vi "TEST.vi"() -> ()   [LabVIEW 2021]
uses:
  Control 4.ctl
  TEST ENNUM.ctl
  <vilib>/Utility/miscctls.llb/LVPointTypeDef.ctl
  Settings page.vi
  Exit Variable.vi
  <vilib>/Instr/_visa.llb/VISA Configure Serial Port (Instr).vi
  <vilib>/Utility/config.llb/Write Key (Double).vi
  <vilib>/Utility/file.llb/Write Delimited Spreadsheet (string).vi
  <vilib>/Utility/config.llb/NI_LVConfig.lvlib
  <userlib>/_OpenG.lib/string/string.llb/openg_string.lvlib
panel:
  out "Boolean":bool
  out "read buffer":string
  out "x/y":dbl
  out "output cluster":T1={"VISA resource name"="COM5", "MODE"="", "PP 1"=0, "PP 2"=0, "PP 3"=0, "PP 4"=0, "PP 5"=0, "PP 6"=0, "PP 7"=0, "PP 8"=0, "PP 9"=0, "PP 10"=0, "CH  PASS  1"=FALSE, "CH  PASS 2"=FALSE, "CH  PASS 3"=FALSE, "CH  PASS 4"=FALSE, "CH  PASS 5"=FALSE, "CH  PASS 6"=FALSE, "CH  PASS 7"=FALSE, "CH  PASS 8"=FALSE, "CH  PASS 9"=FALSE, "CH  PASS 10"=FALSE, "CH  FAIL 1"=FALSE, "CH  FAIL 2"=FALSE, "CH  FAIL 3"=FALSE, "CH  FAIL 4"=FALSE, "CH  FAIL 5"=FALSE, "CH  FAIL 6"=FALSE, "CH  FAIL 7"=FALSE, "CH  FAIL 8"=FALSE, "CH  FAIL 9"=FALSE, "CH  FAIL 10"=FALSE, "RES VALUE 1"=0.0, "RES VALUE 2"=0.0, "RES VALUE 3"=0.0, "RES VALUE 4"=0.0, "RES VALUE 5"=0.0, "RES VALUE 6"=0.0, "RES VALUE 7"=0.0, "RES VALUE 8"=0.0, "RES VALUE 9"=0.0, "RES VALUE 10"=0.0, "SET VALUE 1"=0.0, "SET VALUE 2"=0.0, "SET VALUE 3"=0.0, "SET VALUE 4"=0.0, "SET VALUE 5"=0.0, "SET VALUE 6"=0.0, "SET VALUE 7"=0.0, "SET VALUE 8"=0.0, "SET VALUE 9"=0.0, "SET VALUE 10"=0.0, "TOL 1"=0.0, "TOL 2"=0.0, "TOL 3"=0.0, "TOL 4"=0.0, "TOL 5"=0.0, "TOL 6"=0.0, "TOL 7"=0.0, "TOL 8"=0.0, "TOL 9"=0.0, "TOL 10"=0.0, "START BIT"=0, "CH1 MIN TOL"=0.0, "CH2 MIN TOL "=0.0, "CH3 MIN TOL "=0.0, "CH4 MIN TOL "=0.0, "CH5 MIN TOL "=0.0, "CH6 MIN TOL "=0.0, "CH7 MIN TOL  "=0.0, "CH8 MIN TOL  "=0.0, "CH9 MIN TOL   "=0.0, "CH10 MIN TOL   "=0.0, "CH1 MAX TOL "=0.0, "CH2 MAX TOL  "=0.0, "CH3 MAX TOL  "=0.0, "CH4 MAX TOL "=0.0, "CH5 MAX TOL  "=0.0, "CH6 MAX TOL  "=0.0, "CH7 MAX TOL   "=0.0, "CH8 MAX TOL  "=0.0, "CH9 MAX TOL    "=0.0, "CH10 MAX TOL   "=0.0} {"PP 10" format="%_1f"}
  in  "appended path":path
  out "Printer":bool
  out "Part ID":string
  out "Printer Command":string
  out "TETS TYPE":string
  out "TETS MODE":string
  in  "Exit Button":bool
  in  "SETTINGS BUTTON 2":bool
  out "Communication Status":bool
  out "CH 1 FAIL":bool
  out "CH 10 FAIL":bool
  out "CH 10  PASS":bool
  out "CH 5 FAIL":bool
  out "CH 5 PASS":bool
  out "CH 4 FAIL":bool
  out "CH 4 PASS":bool
  out "CH 9 FAIL":bool
  out "CH 9 PASS":bool
  out "CH 8 FAIL":bool
  out "CH 8 PASS":bool
  out "CH 3 FAIL":bool
  out "CH 3 PASS":bool
  out "CH 2 FAIL":bool
  out "CH 2 PASS":bool
  out "CH 7 FAIL":bool
  out "CH 7 PASS":bool
  out "CH 6 FAIL":bool
  out "CH 6 PASS":bool
  out "CH 1 PASS":bool
  out "CH 10 RES VAL":string
  out "CH 10 STATUS":string
  out "CH 9 RES VAL":string
  out "CH 9 STATUS":string
  out "CH 8 RES VAL":string
  out "CH 8 STATUS":string
  out "CH 7 RES VAL":string
  out "CH 7 STATUS":string
  out "CH 6 RES VAL":string
  out "CH 6 STATUS":string
  out "CH 5 RES VAL":string
  out "CH 5 STATUS":string
  out "CH 4 RES VAL":string
  out "CH 4 STATUS":string
  out "CH 3 RES VAL":string
  out "CH 3 STATUS":string
  out "CH 2 RES VAL":string
  out "CH 2 STATUS":string
  out "Cancel Button":bool
  out "CH 1 RES VAL":string
  out "CH1 STATUS":string
  # "EOL TEST BENCH FOR THERMISTOR"
  # "Communication Status"
  # "Printer Communication Status"
  # "CHANNEL 5"
  # "CHANNEL 3"
  # "CHANNEL 4"
  # "CHANNEL 1"
  # "CHANNEL 2"
  # "STATUS"
  # "STATUS"
  # "STATUS"
  # "STATUS"
  # "STATUS"
  # "k Ohm"
  # "k Ohm"
  # "RESISTANCE VALUE"
  # "RESISTANCE VALUE"
  # "RESISTANCE VALUE"
  # "k Ohm"
  # "RESISTANCE VALUE"
  # "k Ohm"
  # "RESISTANCE VALUE"
  # "k Ohm"
  # "PASS"
  # "FAIL"
  # "PASS"
  # "FAIL"
  # "PASS"
  # "FAIL"
  # "PASS"
  # "FAIL"
  # "PASS"
  # "FAIL"
  # "QR DATA"
  # "CHANNEL 7"
  # "CHANNEL 6"
  # "CHANNEL 10"
  # "CHANNEL 8"
  # "CHANNEL 9"
  # "STATUS"
  # "STATUS"
  # "STATUS"
  # "STATUS"
  # "STATUS"
  # "RESISTANCE VALUE"
  # "RESISTANCE VALUE"
  # "k Ohm"
  # "RESISTANCE VALUE"
  # "Control 4.ctlk Ohm"
  # "RESISTANCE VALUE"
  # "k Ohm"
  # "k Ohm"
  # "RESISTANCE VALUE"
  # "k Ohm"
  # "PASS"
  # "FAIL"
  # "PASS"
  # "FAIL"
  # "PASS"
  # "FAIL"
  # "PASS"
  # "FAIL"
  # "PASS"
  # "FAIL"
  # "MODE :"
  # "TEST TYPE :"
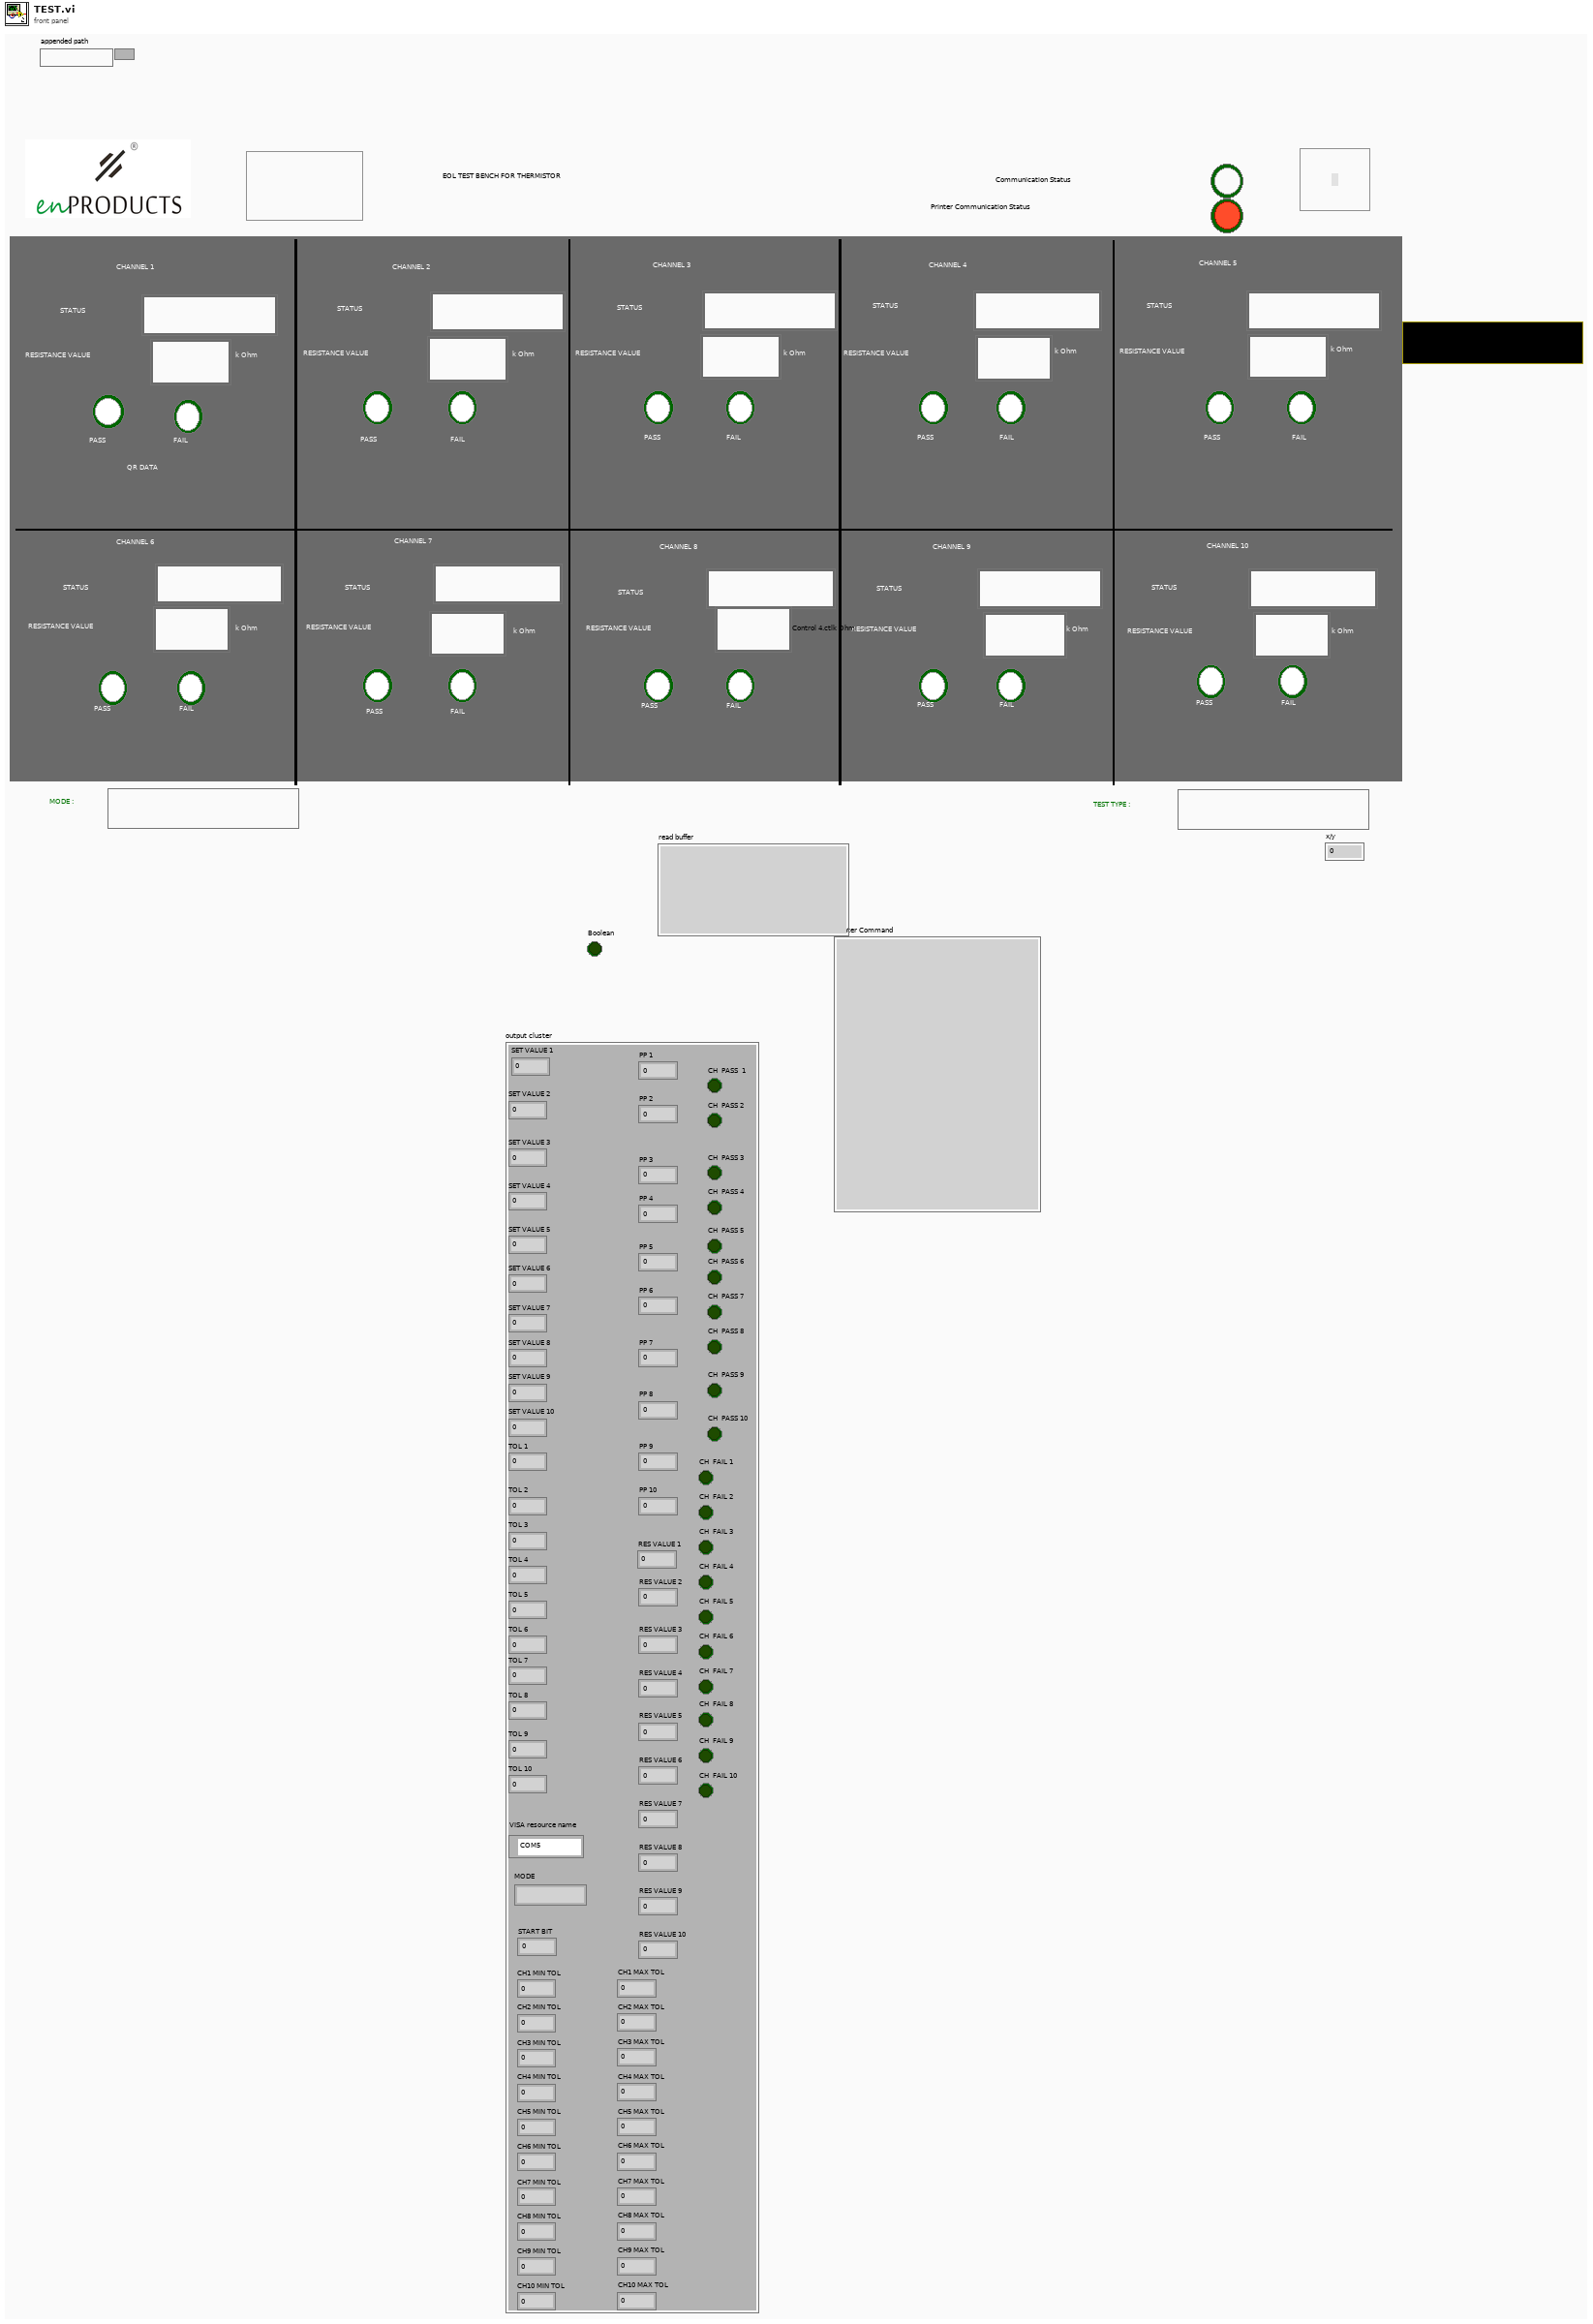
[diagram p1: front panel]
types:
  T1 = typedef "Control 4.ctl" = cluster{"VISA resource name":refnum<visa-resource-name>, "MODE":string, "PP 1":i32, "PP 2":i32, "PP 3":i32, "PP 4":i32, "PP 5":i32, "PP 6":i32, "PP 7":i32, "PP 8":i32, "PP 9":i32, "PP 10":i32, "CH  PASS  1":bool, "CH  PASS 2":bool, "CH  PASS 3":bool, "CH  PASS 4":bool, "CH  PASS 5":bool, "CH  PASS 6":bool, "CH  PASS 7":bool, "CH  PASS 8":bool, "CH  PASS 9":bool, "CH  PASS 10":bool, "CH  FAIL 1":bool, "CH  FAIL 2":bool, "CH  FAIL 3":bool, "CH  FAIL 4":bool, "CH  FAIL 5":bool, "CH  FAIL 6":bool, "CH  FAIL 7":bool, "CH  FAIL 8":bool, "CH  FAIL 9":bool, "CH  FAIL 10":bool, "RES VALUE 1":dbl, "RES VALUE 2":dbl, "RES VALUE 3":dbl, "RES VALUE 4":dbl, "RES VALUE 5":dbl, "RES VALUE 6":dbl, "RES VALUE 7":dbl, "RES VALUE 8":dbl, "RES VALUE 9":dbl, "RES VALUE 10":dbl, "SET VALUE 1":dbl, "SET VALUE 2":dbl, "SET VALUE 3":dbl, "SET VALUE 4":dbl, "SET VALUE 5":dbl, "SET VALUE 6":dbl, "SET VALUE 7":dbl, "SET VALUE 8":dbl, "SET VALUE 9":dbl, "SET VALUE 10":dbl, "TOL 1":dbl, "TOL 2":dbl, "TOL 3":dbl, "TOL 4":dbl, "TOL 5":dbl, "TOL 6":dbl, "TOL 7":dbl, "TOL 8":dbl, "TOL 9":dbl, "TOL 10":dbl, "START BIT":i32, "CH1 MIN TOL":dbl, "CH2 MIN TOL ":dbl, "CH3 MIN TOL ":dbl, "CH4 MIN TOL ":dbl, "CH5 MIN TOL ":dbl, "CH6 MIN TOL ":dbl, "CH7 MIN TOL  ":dbl, "CH8 MIN TOL  ":dbl, "CH9 MIN TOL   ":dbl, "CH10 MIN TOL   ":dbl, "CH1 MAX TOL ":dbl, "CH2 MAX TOL  ":dbl, "CH3 MAX TOL  ":dbl, "CH4 MAX TOL ":dbl, "CH5 MAX TOL  ":dbl, "CH6 MAX TOL  ":dbl, "CH7 MAX TOL   ":dbl, "CH8 MAX TOL  ":dbl, "CH9 MAX TOL    ":dbl, "CH10 MAX TOL   ":dbl}
  T2 = typedef "LVPointTypeDef.ctl" = cluster{"Horizontal":i16, "Vertical":i16}
  T3 = typedef "TEST ENNUM.ctl" = enum16{"TIMEOUT", "INITIALIZE", "CH SELECTION", "VALIDATING", "RESULT", "LED_SEQ", "READY TO PRINT", "REPORT ", "PART PRESENCE CHECKING"}
  T4 = typedef "NI_LVConfig.lvlib/Config Data RefNum.ctl" = refnum<k1>
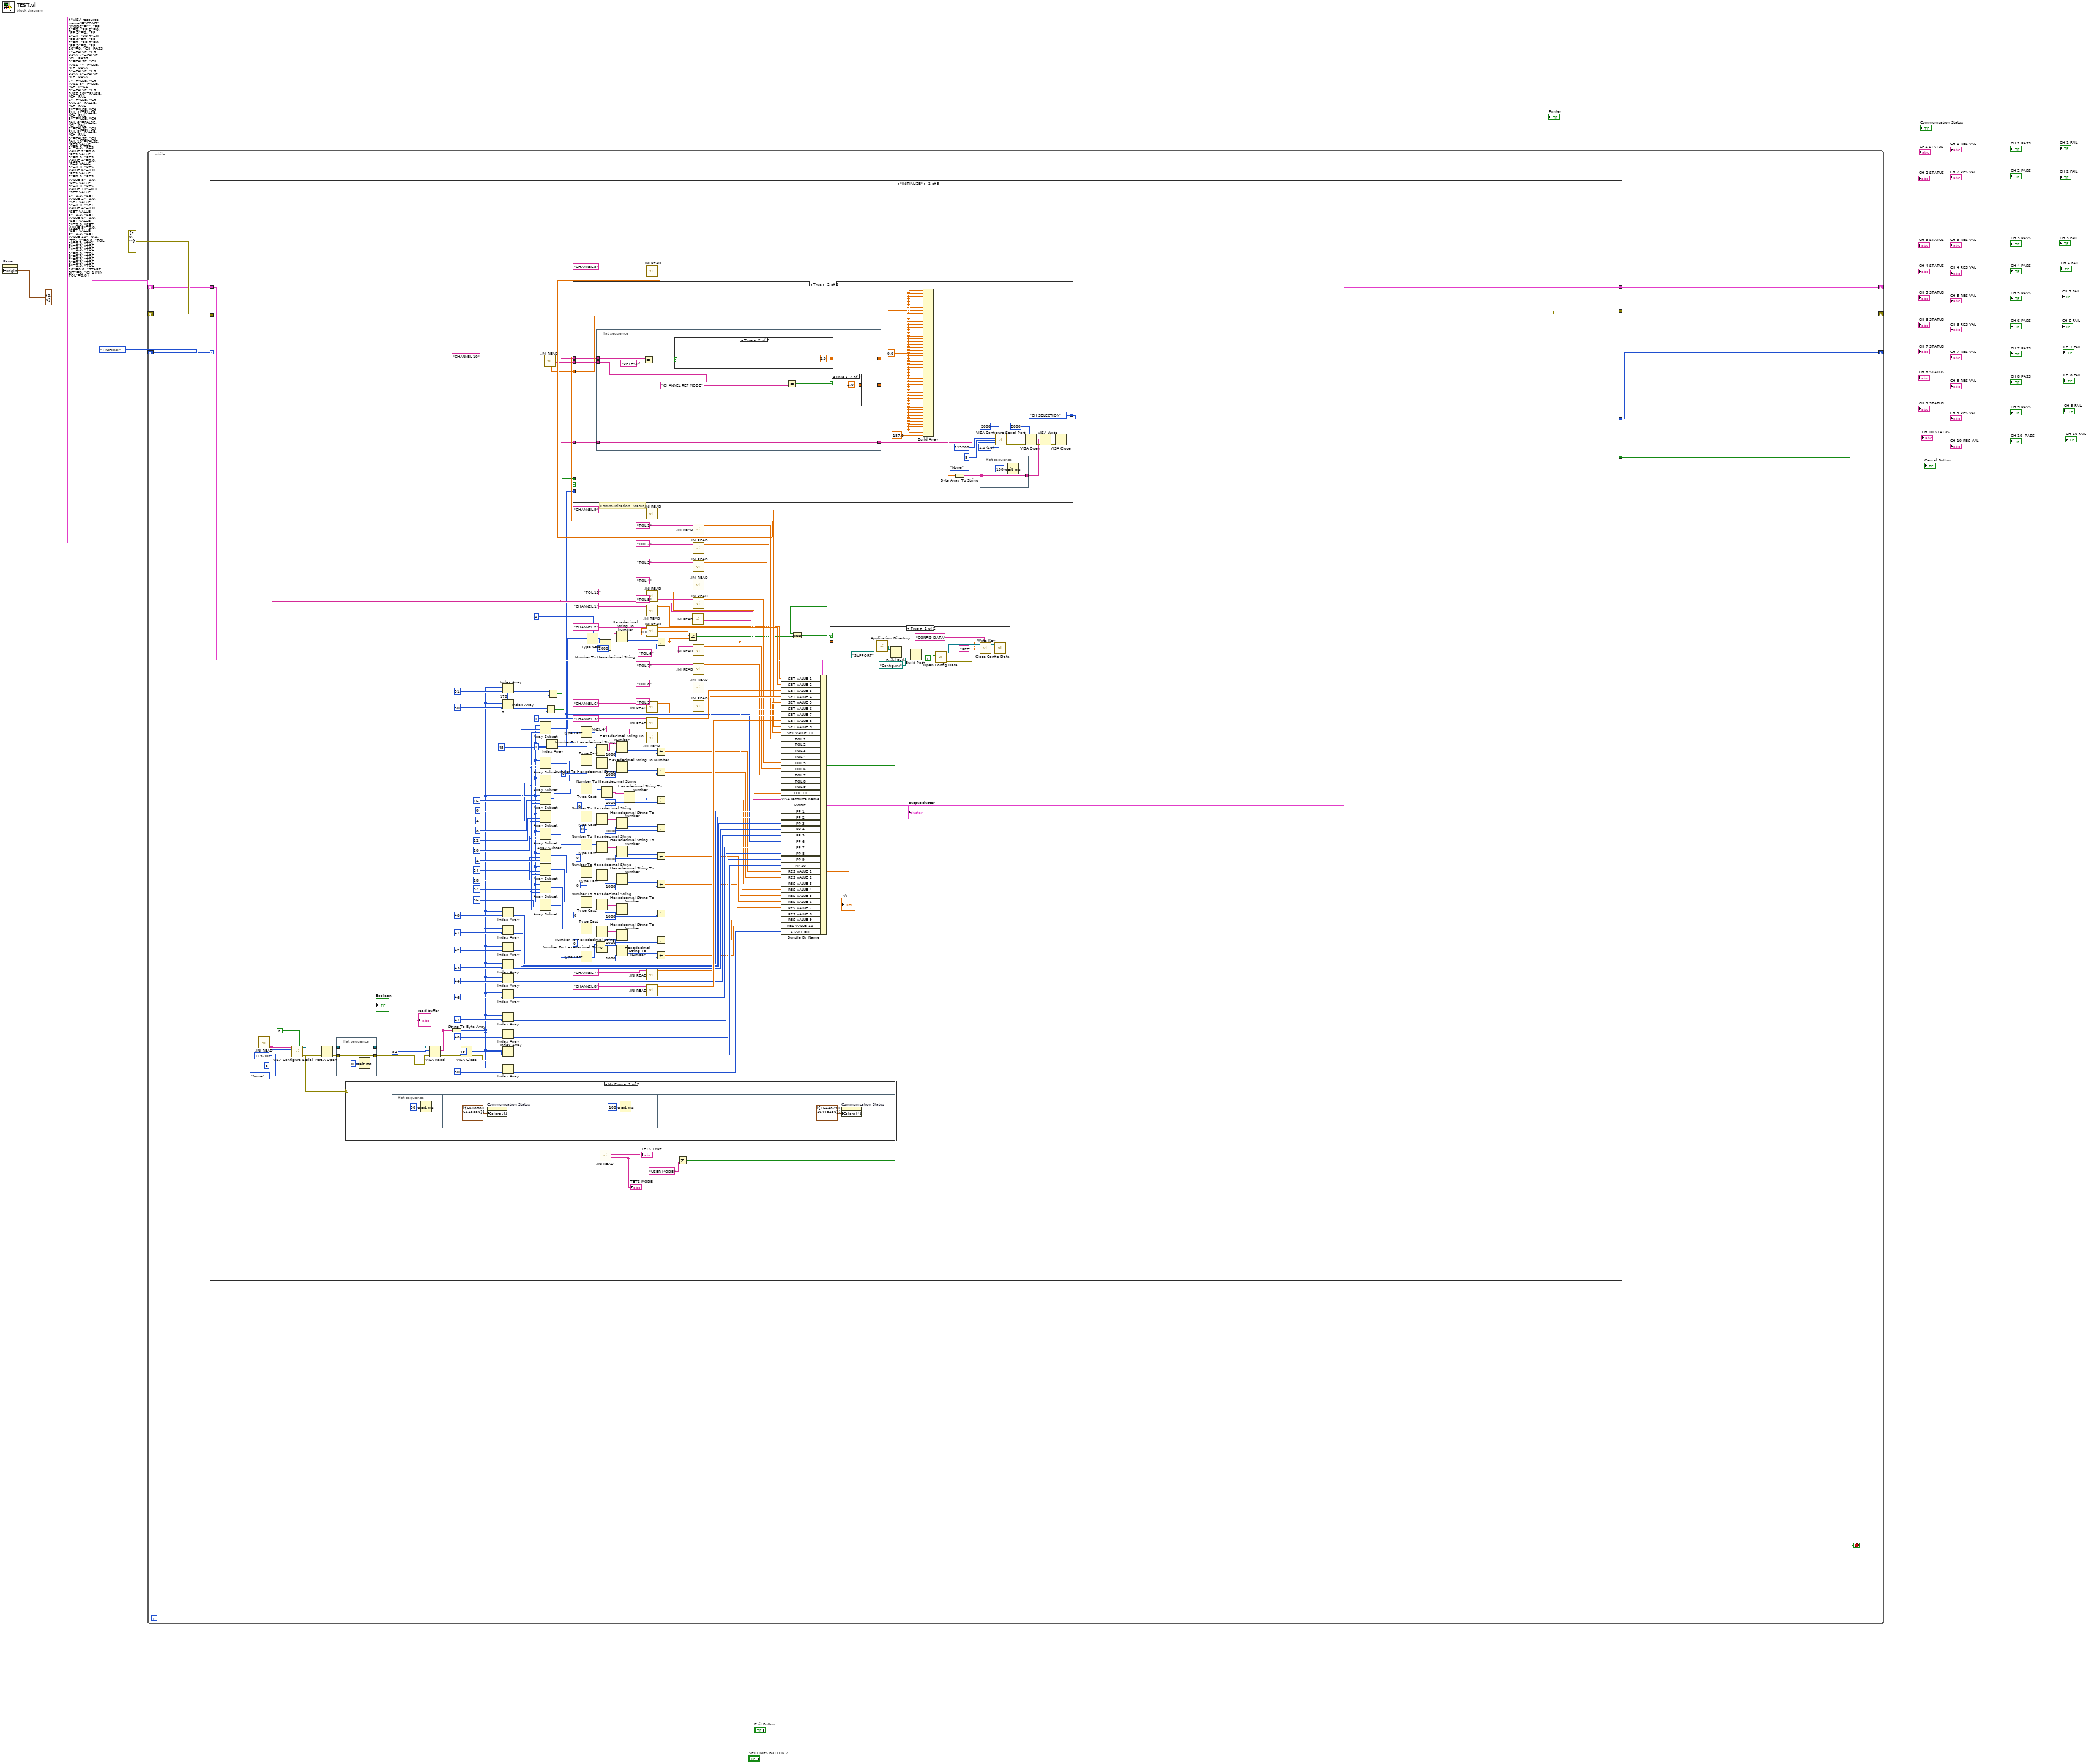
[diagram p0: block diagram]
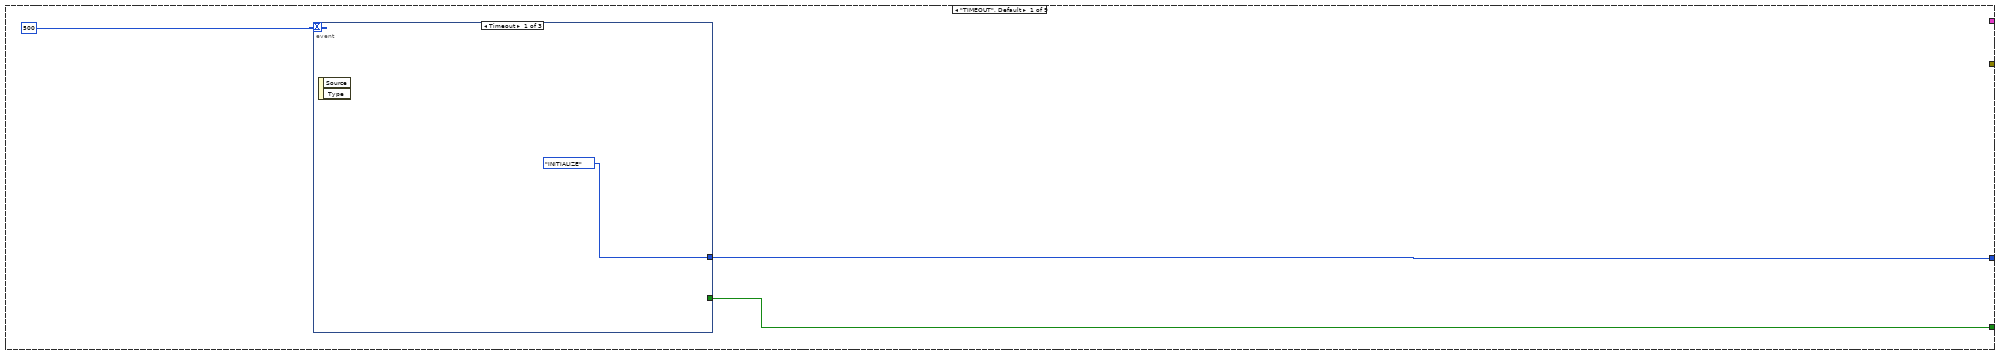
[diagram p2: hidden frame]
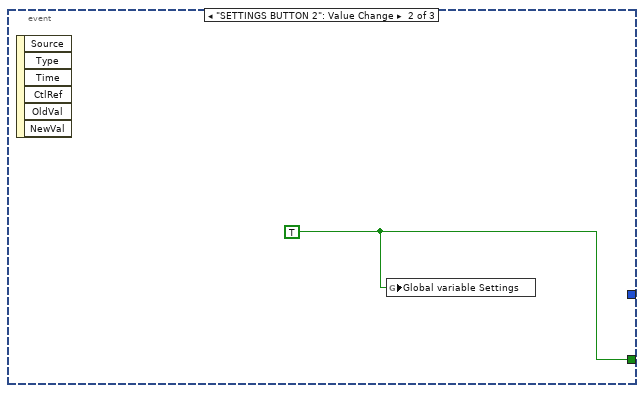
[diagram p3: hidden frame]
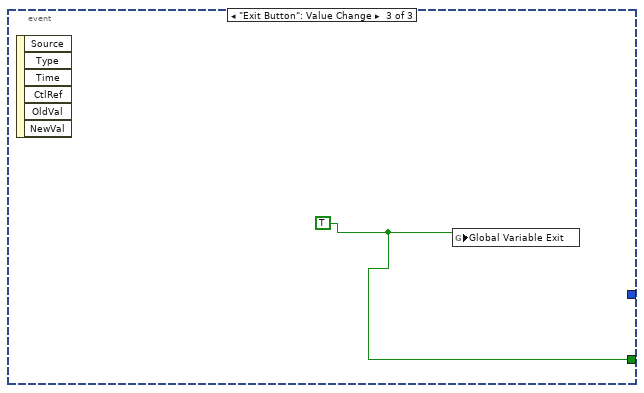
[diagram p4: hidden frame]
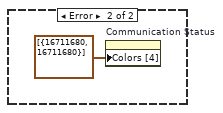
[diagram p6: hidden frame]
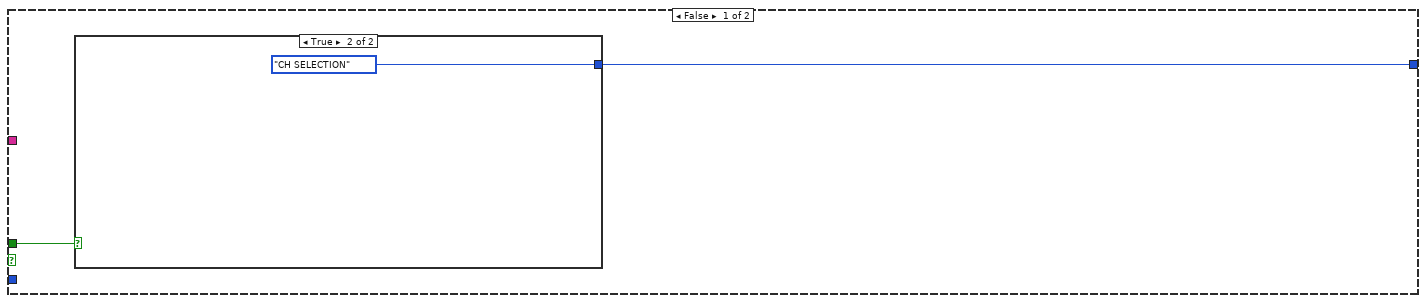
[diagram p7: hidden frame]
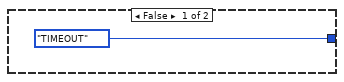
[diagram p8: hidden frame]
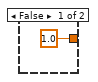
[diagram p9: hidden frame]
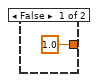
[diagram p10: hidden frame]
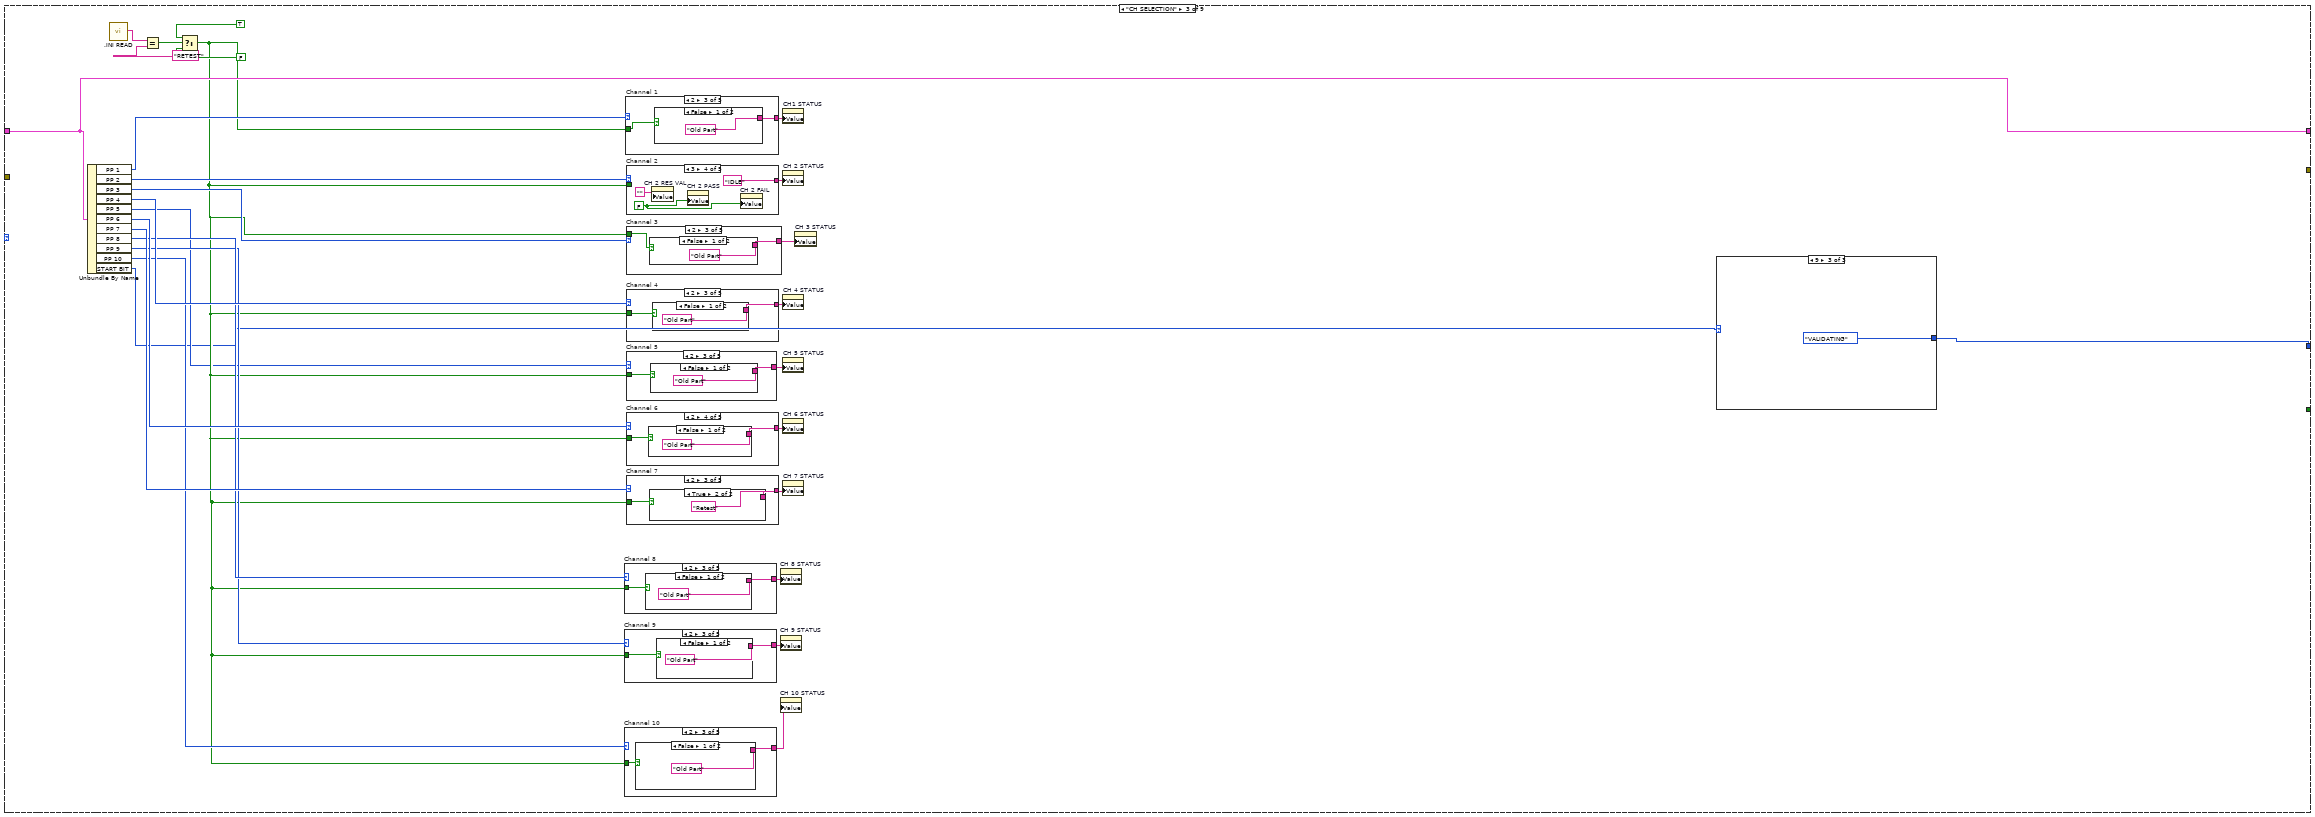
[diagram p11: hidden frame]
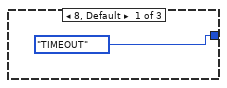
[diagram p12: hidden frame]
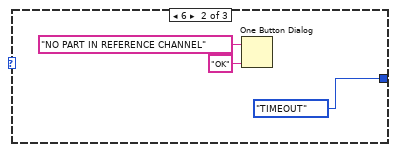
[diagram p13: hidden frame]
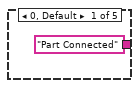
[diagram p14: hidden frame]
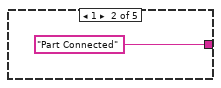
[diagram p15: hidden frame]
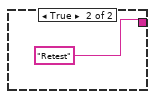
[diagram p16: hidden frame]
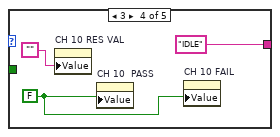
[diagram p17: hidden frame]
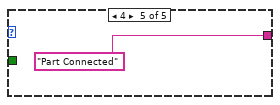
[diagram p18: hidden frame]
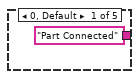
[diagram p19: hidden frame]
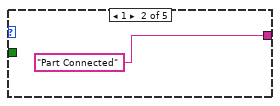
[diagram p20: hidden frame]
diagram:
  n1 = property on="Pane" class="Pane"("Origin"=T2 {"Horizontal"=0, "Vertical"=0}) -> ()  [unwired: 2 in, 2 out]
  n2 = while {
    shift-right: [w10] -> _
    shift-left: TEST_ENNUM."TIMEOUT" -> [w11]
    shift-right: [w9] -> _
    shift-left: T1 {"VISA resource name"="COM5", "MODE"="", "PP 1"=0, "PP 2"=0, "PP 3"=0, "PP 4"=0, "PP 5"=0, "PP 6"=0, "PP 7"=0, "PP 8"=0, "PP 9"=0, "PP 10"=0, "CH  PASS  1"=FALSE, "CH  PASS 2"=FALSE, "CH  PASS 3"=FALSE, "CH  PASS 4"=FALSE, "CH  PASS 5"=FALSE, "CH  PASS 6"=FALSE, "CH  PASS 7"=FALSE, "CH  PASS 8"=FALSE, "CH  PASS 9"=FALSE, "CH  PASS 10"=FALSE, "CH  FAIL 1"=FALSE, "CH  FAIL 2"=FALSE, "CH  FAIL 3"=FALSE, "CH  FAIL 4"=FALSE, "CH  FAIL 5"=FALSE, "CH  FAIL 6"=FALSE, "CH  FAIL 7"=FALSE, "CH  FAIL 8"=FALSE, "CH  FAIL 9"=FALSE, "CH  FAIL 10"=FALSE, "RES VALUE 1"=0.0, "RES VALUE 2"=0.0, "RES VALUE 3"=0.0, "RES VALUE 4"=0.0, "RES VALUE 5"=0.0, "RES VALUE 6"=0.0, "RES VALUE 7"=0.0, "RES VALUE 8"=0.0, "RES VALUE 9"=0.0, "RES VALUE 10"=0.0, "SET VALUE 1"=0.0, "SET VALUE 2"=0.0, "SET VALUE 3"=0.0, "SET VALUE 4"=0.0, "SET VALUE 5"=0.0, "SET VALUE 6"=0.0, "SET VALUE 7"=0.0, "SET VALUE 8"=0.0, "SET VALUE 9"=0.0, "SET VALUE 10"=0.0, "TOL 1"=0.0, "TOL 2"=0.0, "TOL 3"=0.0, "TOL 4"=0.0, "TOL 5"=0.0, "TOL 6"=0.0, "TOL 7"=0.0, "TOL 8"=0.0, "TOL 9"=0.0, "TOL 10"=0.0, "START BIT"=0, "CH1 MIN TOL"=0.0, "CH2 MIN TOL "=0.0, "CH3 MIN TOL "=0.0, "CH4 MIN TOL "=0.0, "CH5 MIN TOL "=0.0, "CH6 MIN TOL "=0.0, "CH7 MIN TOL  "=0.0, "CH8 MIN TOL  "=0.0, "CH9 MIN TOL   "=0.0, "CH10 MIN TOL   "=0.0, "CH1 MAX TOL "=0.0, "CH2 MAX TOL  "=0.0, "CH3 MAX TOL  "=0.0, "CH4 MAX TOL "=0.0, "CH5 MAX TOL  "=0.0, "CH6 MAX TOL  "=0.0, "CH7 MAX TOL   "=0.0, "CH8 MAX TOL  "=0.0, "CH9 MAX TOL    "=0.0, "CH10 MAX TOL   "=0.0} ("Cluster") -> [w7]
    shift-right: [w8] -> _
    shift-left: errorcluster {"status"=FALSE, "code"=0, "source"=""} ("error out") -> [w6]
    stop <- w5 stop-if-true
    n3 = case shown="\"INITIALIZE\"" w11 {
      tunnel: [w13 w55 w265 TEST_ENNUM."RESULT" TEST_ENNUM."LED_SEQ" TEST_ENNUM."READY TO PRINT" TEST_ENNUM."REPORT " TEST_ENNUM."TIMEOUT" _] -> w10
      tunnel: w7 -> [_ w139 w274 w421 w641 w860 w1021 w1032 _]
      tunnel: [_ w140 w274 w534 w641 w860 _ _ _] -> w9
      tunnel: [_ w59 _ _ _ w858 _ _ _] -> w8
      tunnel: w6 -> [_ _ _ _ _ _ _ _ _]
      tunnel: [w12 _ _ _ _ _ _ _ _] -> w5
      frame "TIMEOUT", Default {
        n4 = event shown="[0] Timeout" {
          selector: _ -> [_ _ _]
          dyn-events: _ -> [_ _ _]
          timeout: 500 -> [_ _ _]
          tunnel: [_ w16 w17] -> w12
          tunnel: [TEST_ENNUM."INITIALIZE" _ _] -> w13
          event Timeout {
            n5 = event-data() -> ()  [unwired: 1 in, 2 out]
          }
          event "SETTINGS BUTTON 2": Value Change {
            w16 = TRUE
            n6 = event-data() -> ()  [unwired: 1 in, 6 out]
            n7 = global write "Settings page.vi" "Global variable Settings"(w16) -> ()
          }
          event "Exit Button": Value Change {
            w17 = TRUE
            n8 = event-data() -> ()  [unwired: 1 in, 6 out]
            n9 = global write "Exit Variable.vi" "Global Variable Exit"(w17) -> ()
          }
        }
      }
      frame "INITIALIZE" {
        w137 = 4 ("length")
        # "Communication  Status"
        n10 = call ".INI READ.vi"() -> ("COM"=w56:string)  [unwired: 4 in, 7 out]
        n11 = call-poly "VISA Configure Serial Port"("VISA resource name"=w56, "Enable Termination\nChar (T)"=FALSE ("Enable Termination\nChar (T)"), "baud rate (9600)"=u32 115200, "data bits (8)"=u16 8, "parity (0:none)"=enum16{"None", "Odd", "Even", "Mark", "Space"}."None") -> ("VISA resource name out"=w47:refnum<visa-resource-name>, "error out"=w61:errorcluster)  [unwired: 9 in]
        n12 = VISA Open(error in (no error)=w61, VISA resource name=w47) -> (VISA resource name=w42:refnum<visa-resource-name>, error out=w44:errorcluster)  [unwired: 3 in]
        n13 = flat-sequence {
          tunnel: [w215] -> w21
          tunnel: w44 -> [w215]
          tunnel: [w214] -> w43
          tunnel: w42 -> [w214]
          frame #0 {
            n14 = Wait (ms)(milliseconds to wait=u32 0) -> ()  [unwired: 1 out]
          }
        }
        n15 = case shown="No Error" w61 {
          frame No Error {
            n16 = flat-sequence {
              frame #0 {
                n17 = Wait (ms)(milliseconds to wait=u32 50) -> ()  [unwired: 1 out]
              }
              frame #1 {
                n18 = property on="Communication Status" class="Bool (strict)"("Colors [4]"=cluster{u32, u32}[] [{6618880, 6618880}]) -> ()  [unwired: 2 in, 2 out]
              }
              frame #2 {
                n19 = Wait (ms)(milliseconds to wait=u32 100) -> ()  [unwired: 1 out]
              }
              frame #3 {
                n20 = property on="Communication Status" class="Bool (strict)"("Colors [4]"=cluster{u32, u32}[] [{16448250, 16448250}]) -> ()  [unwired: 2 in, 2 out]
              }
            }
          }
          frame Error {
            n21 = property on="Communication Status" class="Bool (strict)"("Colors [4]"=cluster{u32, u32}[] [{16711680, 16711680}]) -> ()  [unwired: 2 in, 2 out]
          }
        }
        n22 = VISA Read(VISA resource name=w43, byte count=u32 52, error in (no error)=w21) -> (VISA resource name out=w19:refnum<visa-resource-name>, read buffer=w20:string, error out=w18:errorcluster)  [unwired: 1 out]
        "read buffer" <- w20
        n23 = String To Byte Array(string=w20) -> (unsigned byte array=w34:u8[])
        n24 = VISA Close(VISA resource name=w19, error in (no error)=w18) -> (error out=w59:errorcluster)
        n25 = Index Array(array=w34, index=51) -> (element=w57:u8)
        n26 = Index Array(array=w34, index=50) -> (element=w52:u8)
        n27 = Index Array(array=w34, index=40) -> (element=w149:u8)
        n28 = Index Array(array=w34, index=41) -> (element=w148:u8)
        n29 = Index Array(array=w34, index=42) -> (element=w147:u8)
        n30 = Index Array(array=w34, index=43) -> (element=w146:u8)
        n31 = Index Array(array=w34, index=44) -> (element=w145:u8)
        n32 = Index Array(array=w34, index=46) -> (element=w144:u8)
        n33 = Index Array(array=w34, index=47) -> (element=w143:u8)
        n34 = Index Array(array=w34, index=48) -> (element=w142:u8)
        n35 = Index Array(array=w34, index=49) -> (element=w141:u8)
        n36 = Index Array(array=w34, index=50) -> (element=w60:u8)
        n37 = Array Subset(array=w34, index=16, length=w137) -> (w109:u8[])
        n38 = Array Subset(array=w34, index=0, length=w137) -> (w24:u8[])
        n39 = Array Subset(array=w34, index=4, length=w137) -> (w116:u8[])
        n40 = Array Subset(array=w34, index=8, length=w137) -> (w23:u8[])
        n41 = Array Subset(array=w34, index=12, length=w137) -> (w112:u8[])
        n42 = Array Subset(array=w34, index=20, length=w137) -> (w106:u8[])
        n43 = Array Subset(array=w34, index=24, length=w137) -> (w103:u8[])
        n44 = Array Subset(array=w34, index=28, length=w137) -> (w100:u8[])
        n45 = Array Subset(array=w34, index=32, length=w137) -> (w97:u8[])
        n46 = Array Subset(array=w34, index=36, length=w137) -> (w94:u8[])
        n47 = call ".INI READ.vi"("KEY"="CHANNEL 10") -> ("MODE"=w30:string, "TEST MODE"=w29:string, "OUT"=w181:dbl, "TIME"=w31:dbl)  [unwired: 3 in, 4 out]
        n48 = Equal?(x=w52, y=u8 8) -> (x = y?=w50:bool)
        n49 = Index Array(array=w34, index=45) -> (element=w32:u8)
        n50 = Equal?(x=w57, y=u8 170) -> (x = y?=w53:bool)
        n51 = case shown="True" w50 {
          tunnel: w56 -> [_ w229]
          tunnel: [w221 TEST_ENNUM."CH SELECTION"] -> w55
          tunnel: w53 -> [w222 _]
          tunnel: w32 -> [_ _]
          tunnel: w30 -> [_ w227]
          tunnel: w31 -> [_ w226]
          tunnel: w29 -> [_ w225]
          frame False {
            n52 = case shown="True" w222 {
              tunnel: [TEST_ENNUM."TIMEOUT" TEST_ENNUM."CH SELECTION"] -> w221
              frame False {
              }
              frame True {
              }
            }
          }
          frame True {
            w242 = u16 10 items=["1.0"=10, "1.5"=15, "2.0"=20] ("stop bits (10: 1 bit)")
            w233 = 0.0 ("element")
            n53 = flat-sequence {
              tunnel: [w256] -> w231
              tunnel: [w253] -> w230
              tunnel: w229 -> [w252]
              tunnel: [w252] -> w228
              tunnel: w227 -> [w251]
              tunnel: w225 -> [w250]
              frame #0 {
                n54 = Equal?(x=w250, y="RETEST") -> (x = y?=w257:bool)
                n55 = case shown="True" w257 {
                  tunnel: [1.0 ("element") 2.0 ("element")] -> w256
                  frame False {
                  }
                  frame True {
                  }
                }
                n56 = Equal?(x=w251, y="CHANNEL REF MODE") -> (x = y?=w254:bool)
                n57 = case shown="True" w254 {
                  tunnel: [1.0 ("element") 2.0 ("element")] -> w253
                  frame False {
                  }
                  frame True {
                  }
                }
              }
            }
            n58 = Build Array(w233, w233, w233, w233, w233, w233, w231, w230, w233, w226, w233, w233, w233, w233, w233, w233, w233, w233, w233, w233, w233, w233, w233, w233, w233, w233, w233, w233, w233, w233, w233, w233, w233, w233, w233, w233, w233, w233, w233, w233, w233, w233, w233, w233, w233, w233, w233, w233, w233, w233, w233, 187.0 ("element")) -> (w249:dbl[])
            n59 = Byte Array To String(unsigned byte array=w249) -> (string=w235:string)
            n60 = flat-sequence {
              tunnel: w235 -> [w264]
              tunnel: [w264] -> w234
              frame #0 {
                n61 = Wait (ms)(milliseconds to wait=u32 100) -> ()  [unwired: 1 out]
              }
            }
            n62 = call-poly "VISA Configure Serial Port"("VISA resource name"=w228, "timeout (10sec)"=u32 2000, "baud rate (9600)"=u32 115200, "data bits (8)"=u16 8, "parity (0:none)"=enum16{"None", "Odd", "Even", "Mark", "Space"}."None", "stop bits (10: 1 bit)"=w242) -> ("VISA resource name out"=w248:refnum<visa-resource-name>, "error out"=w247:errorcluster)  [unwired: 8 in]
            n63 = VISA Open(timeout (0)=u32 2000 ("VISA Open timeout (0)"), error in (no error)=w247, VISA resource name=w248) -> (VISA resource name=w241:refnum<visa-resource-name>, error out=w240:errorcluster)  [unwired: 2 in]
            n64 = VISA Write(VISA resource name=w241, write buffer=w234, error in (no error)=w240) -> (VISA resource name out=w238:refnum<visa-resource-name>, error out=w237:errorcluster)  [unwired: 1 out]
            n65 = VISA Close(VISA resource name=w238, error in (no error)=w237) -> ()  [unwired: 1 out]
          }
        }
        n66 = Type Cast(type=0 ("index"), x=w24) -> (*(type *) &x=w118:i32)
        n67 = Type Cast(type=0 ("index"), x=w116) -> (*(type *) &x=w115:i32)
        n68 = Type Cast(type=0 ("index"), x=w23) -> (*(type *) &x=w22:i32)
        n69 = Type Cast(type=0 ("index"), x=w112) -> (*(type *) &x=w111:i32)
        n70 = Type Cast(type=0 ("index"), x=w106) -> (*(type *) &x=w105:i32)
        n71 = Type Cast(type=0 ("index"), x=w103) -> (*(type *) &x=w102:i32)
        n72 = Type Cast(type=0 ("index"), x=w100) -> (*(type *) &x=w99:i32)
        n73 = Type Cast(type=0 ("index"), x=w97) -> (*(type *) &x=w96:i32)
        n74 = Type Cast(type=0 ("index"), x=w94) -> (*(type *) &x=w93:i32)
        n75 = Type Cast(type=0 ("index"), x=w109) -> (*(type *) &x=w108:i32)
        n76 = Number To Hexadecimal String(2:w118) -> (0:w117:string)  [unwired: 1 in]
        n77 = Number To Hexadecimal String(2:w115) -> (0:w114:string)  [unwired: 1 in]
        n78 = Number To Hexadecimal String(2:w111) -> (0:w110:string)  [unwired: 1 in]
        n79 = Number To Hexadecimal String(2:w105) -> (0:w104:string)  [unwired: 1 in]
        n80 = Number To Hexadecimal String(2:w102) -> (0:w101:string)  [unwired: 1 in]
        n81 = Number To Hexadecimal String(2:w99) -> (0:w98:string)  [unwired: 1 in]
        n82 = Number To Hexadecimal String(2:w96) -> (0:w95:string)  [unwired: 1 in]
        n83 = Number To Hexadecimal String(2:w93) -> (0:w92:string)  [unwired: 1 in]
        n84 = Number To Hexadecimal String(2:w108) -> (0:w107:string)  [unwired: 1 in]
        n85 = call ".INI READ.vi"() -> ("MODE"=w28:string, "TEST MODE"=→"TETS TYPE":string)  [unwired: 4 in, 6 out]
        "TETS MODE" <- w28
        n86 = Number To Hexadecimal String(2:w22) -> (0:w113:string)  [unwired: 1 in]
        n87 = Hexadecimal String To Number(string=w107) -> (number=w80:u32)  [unwired: 2 in, 1 out]
        n88 = Hexadecimal String To Number(string=w117) -> (number=w91:u32)  [unwired: 2 in, 1 out]
        n89 = Hexadecimal String To Number(string=w114) -> (number=w88:u32)  [unwired: 2 in, 1 out]
        n90 = Hexadecimal String To Number(string=w110) -> (number=w83:u32)  [unwired: 2 in, 1 out]
        n91 = Hexadecimal String To Number(string=w104) -> (number=w65:u32)  [unwired: 2 in, 1 out]
        n92 = Hexadecimal String To Number(string=w101) -> (number=w77:u32)  [unwired: 2 in, 1 out]
        n93 = Hexadecimal String To Number(string=w98) -> (number=w74:u32)  [unwired: 2 in, 1 out]
        n94 = Hexadecimal String To Number(string=w95) -> (number=w71:u32)  [unwired: 2 in, 1 out]
        n95 = Hexadecimal String To Number(string=w92) -> (number=w68:u32)  [unwired: 2 in, 1 out]
        n96 = Hexadecimal String To Number(string=w113) -> (number=w86:u32)  [unwired: 2 in, 1 out]
        n97 = call ".INI READ.vi"("KEY"="CHANNEL 5") -> ("OUT"=w186:dbl)  [unwired: 3 in, 7 out]
        n98 = call ".INI READ.vi"("KEY"="CHANNEL 9") -> ("OUT"=w182:dbl)  [unwired: 3 in, 7 out]
        n99 = call ".INI READ.vi"("KEY"="TOL 10") -> ("OUT"=w161:dbl)  [unwired: 3 in, 7 out]
        n100 = call ".INI READ.vi"("KEY"="CHANNEL 1") -> ("OUT"=w39:dbl)  [unwired: 3 in, 7 out]
        n101 = call ".INI READ.vi"("KEY"="CHANNEL 2") -> ("OUT"=w189:dbl)  [unwired: 3 in, 7 out]
        n102 = call ".INI READ.vi"("KEY"="CHANNEL 6") -> ("OUT"=w185:dbl)  [unwired: 3 in, 7 out]
        n103 = call ".INI READ.vi"("KEY"="CHANNEL 3") -> ("OUT"=w188:dbl)  [unwired: 3 in, 7 out]
        n104 = call ".INI READ.vi"("KEY"="CHANNEL 4") -> ("OUT"=w187:dbl)  [unwired: 3 in, 7 out]
        n105 = call ".INI READ.vi"("KEY"="CHANNEL 7") -> ("OUT"=w184:dbl)  [unwired: 3 in, 7 out]
        n106 = call ".INI READ.vi"("KEY"="CHANNEL 8") -> ("OUT"=w183:dbl)  [unwired: 3 in, 7 out]
        n107 = Divide(x=w91, y=u32 1000) -> (x/y=w26:dbl)
        "x/y" <- w26
        n108 = Divide(x=w88, y=u32 1000) -> (x/y=w87:dbl)
        n109 = Divide(x=w86, y=u32 1000) -> (x/y=w84:dbl)
        n110 = Divide(x=w83, y=u32 1000) -> (x/y=w81:dbl)
        n111 = Divide(x=w65, y=u32 1000) -> (x/y=w78:dbl)
        n112 = Divide(x=w77, y=u32 1000) -> (x/y=w75:dbl)
        n113 = Divide(x=w74, y=u32 1000) -> (x/y=w72:dbl)
        n114 = Divide(x=w71, y=u32 1000) -> (x/y=w69:dbl)
        n115 = Divide(x=w68, y=u32 1000) -> (x/y=w63:dbl)
        n116 = Divide(x=w80, y=u32 1000) -> (x/y=w33:dbl)
        n117 = Not Equal?(x=w28, y="USER MODE") -> (x != y?=w36:bool)
        n118 = Not Equal?(x=0.0, y=w33) -> (x != y?=w37:bool)
        n119 = call ".INI READ.vi"() -> ("MODE"=w160:string)  [unwired: 4 in, 7 out]
        n120 = call ".INI READ.vi"("KEY"="TOL 1") -> ("OUT"=w170:dbl)  [unwired: 3 in, 7 out]
        n121 = call ".INI READ.vi"("KEY"="TOL 2") -> ("OUT"=w169:dbl)  [unwired: 3 in, 7 out]
        n122 = call ".INI READ.vi"("KEY"="TOL 3") -> ("OUT"=w168:dbl)  [unwired: 3 in, 7 out]
        n123 = call ".INI READ.vi"("KEY"="TOL 4") -> ("OUT"=w167:dbl)  [unwired: 3 in, 7 out]
        n124 = call ".INI READ.vi"("KEY"="TOL 5") -> ("OUT"=w166:dbl)  [unwired: 3 in, 7 out]
        n125 = call ".INI READ.vi"("KEY"="TOL 6") -> ("OUT"=w165:dbl)  [unwired: 3 in, 7 out]
        n126 = call ".INI READ.vi"("KEY"="TOL 7") -> ("OUT"=w164:dbl)  [unwired: 3 in, 7 out]
        n127 = call ".INI READ.vi"("KEY"="TOL 8") -> ("OUT"=w163:dbl)  [unwired: 3 in, 7 out]
        n128 = call ".INI READ.vi"("KEY"="TOL 9") -> ("OUT"=w162:dbl)  [unwired: 3 in, 7 out]
        n129 = Bundle By Name(cluster=w139, "SET VALUE 1"=w39, "SET VALUE 2"=w189, "SET VALUE 3"=w188, "SET VALUE 4"=w187, "SET VALUE 5"=w186, "SET VALUE 6"=w185, "SET VALUE 7"=w184, "SET VALUE 8"=w183, "SET VALUE 9"=w182, "SET VALUE 10"=w181, "TOL 1"=w170, "TOL 2"=w169, "TOL 3"=w168, "TOL 4"=w167, "TOL 5"=w166, "TOL 6"=w165, "TOL 7"=w164, "TOL 8"=w163, "TOL 9"=w162, "TOL 10"=w161, "VISA resource name"=w56, "MODE"=w160, "PP 1"=w149, "PP 2"=w148, "PP 3"=w147, "PP 4"=w146, "PP 5"=w145, "PP 6"=w32, "PP 7"=w144, "PP 8"=w143, "PP 9"=w142, "PP 10"=w141, "RES VALUE 1"=w26, "RES VALUE 2"=w87, "RES VALUE 3"=w84, "RES VALUE 4"=w81, "RES VALUE 5"=w33, "RES VALUE 6"=w78, "RES VALUE 7"=w75, "RES VALUE 8"=w72, "RES VALUE 9"=w69, "RES VALUE 10"=w63, "START BIT"=w60) -> (w140:T1)
        "output cluster" <- w140
        n130 = And(x=w36, y=w37) -> (x .and. y?=w35:bool)
        n131 = case shown="True" w35 {
          tunnel: w33 -> [_ w200]
          frame False {
          }
          frame True {
            n132 = call <vilib>:"Application Directory.vi"() -> ("Application Directory"=w211:path)
            n133 = Build Path(base path=w211, name or relative path=path "SUPPORT") -> (appended path=w212:path)
            n134 = Build Path(base path=w212, name or relative path=path "Config.ini") -> (appended path=w208:path)
            n135 = call <vilib>:"Open Config Data.vi"("create file if necessary (T)"=TRUE, "configuration file path"=w208) -> ("error out"=w201:errorcluster, "refnum"=w206:T4)  [unwired: 7 in, 1 out]
            n136 = call-poly <vilib>:"Write Key.vi"("section"="CONFIG DATA", "error in (no error)"=w201, "value"=w200, "key"="REF", "refnum"=w206) -> ("error out"=w202:errorcluster, "refnum out"=w203:T4)  [unwired: 4 in, 1 out]
            n137 = call <vilib>:"Close Config Data.vi"("error in (no error)"=w202, "refnum"=w203) -> ()  [unwired: 8 in, 2 out]
          }
        }
      }
      frame "CH SELECTION" {
        n138 = Unbundle By Name(w274) -> ("PP 1"=w293:i32, "PP 2"=w282:i32, "PP 3"=w281:i32, "PP 4"=w280:i32, "PP 5"=w267:i32, "PP 6"=w279:i32, "PP 7"=w278:i32, "PP 8"=w277:i32, "PP 9"=w276:i32, "PP 10"=w275:i32, "START BIT"=w266:i32)
        n139 = call ".INI READ.vi"() -> ("TEST MODE"=w273:string)  [unwired: 4 in, 7 out]
        n140 = Equal?(x=w273, y="RETEST") -> (x = y?=w271:bool)
        n141 = Select(t=TRUE, s=w271, f=FALSE) -> (s? t:f=w268:bool)
        n142 = case "Channel 8" shown="2" w277 {
          tunnel: ["Part Connected" "Part Connected" w322 "IDLE" "Part Conected"] -> w285
          tunnel: w268 -> [_ _ w321 _ _]
          frame 0, Default {
          }
          frame 1 {
          }
          frame 2 {
            n143 = case shown="False" w321 {
              tunnel: ["Old Part" "Retest"] -> w322
              frame False {
              }
              frame True {
              }
            }
          }
          frame 3 {
            w326 = FALSE
            n144 = property on="CH 8 RES VAL" class="Str"("Value"="") -> ()  [unwired: 2 in, 2 out]
            n145 = property on="CH 8 PASS" class="Bool (strict)"("Value"=w326) -> ()  [unwired: 2 in, 2 out]
            n146 = property on="CH 8 FAIL" class="Bool (strict)"("Value"=w326) -> ()  [unwired: 2 in, 2 out]
          }
          frame 4 {
          }
        }
        n147 = case "Channel 9" shown="2" w276 {
          tunnel: ["Part Connected" "Part Connected" w312 "IDLE" "Part Connected"] -> w284
          tunnel: w268 -> [_ _ w311 _ _]
          frame 0, Default {
          }
          frame 1 {
          }
          frame 2 {
            n148 = case shown="False" w311 {
              tunnel: ["Old Part" "Retest"] -> w312
              frame False {
              }
              frame True {
              }
            }
          }
          frame 3 {
            w316 = FALSE
            n149 = property on="CH 9 RES VAL" class="Str"("Value"="") -> ()  [unwired: 2 in, 2 out]
            n150 = property on="CH 9 PASS" class="Bool (strict)"("Value"=w316) -> ()  [unwired: 2 in, 2 out]
            n151 = property on="CH 9 FAIL" class="Bool (strict)"("Value"=w316) -> ()  [unwired: 2 in, 2 out]
          }
          frame 4 {
          }
        }
        n152 = case "Channel 10" shown="2" w275 {
          tunnel: ["Part Connected" "Part Connected" w302 "IDLE" "Part Connected"] -> w283
          tunnel: w268 -> [_ _ w301 _ _]
          frame 0, Default {
          }
          frame 1 {
          }
          frame 2 {
            n153 = case shown="False" w301 {
              tunnel: ["Old Part" "Retest"] -> w302
              frame False {
              }
              frame True {
              }
            }
          }
          frame 3 {
            w306 = FALSE
            n154 = property on="CH 10 RES VAL" class="Str"("Value"="") -> ()  [unwired: 2 in, 2 out]
            n155 = property on="CH 10  PASS" class="Bool (strict)"("Value"=w306) -> ()  [unwired: 2 in, 2 out]
            n156 = property on="CH 10 FAIL" class="Bool (strict)"("Value"=w306) -> ()  [unwired: 2 in, 2 out]
          }
          frame 4 {
          }
        }
        n157 = case "Channel 1" shown="2" w293 {
          tunnel: ["Part Connected" "Part Connected" w392 "IDLE" "Part Connected"] -> w292
          tunnel: w268 -> [_ _ w391 _ _]
          frame 0, Default {
          }
          frame 1 {
          }
          frame 2 {
            n158 = case shown="False" w391 {
              tunnel: ["Old Part" "Retest"] -> w392
              frame False {
              }
              frame True {
              }
            }
          }
          frame 3 {
            w396 = FALSE
            n159 = property on="CH 1 RES VAL" class="Str"("Value"="") -> ()  [unwired: 2 in, 2 out]
            n160 = property on="CH 1 PASS" class="Bool (strict)"("Value"=w396) -> ()  [unwired: 2 in, 2 out]
            n161 = property on="CH 1 FAIL" class="Bool (strict)"("Value"=w396) -> ()  [unwired: 2 in, 2 out]
          }
          frame 4 {
          }
        }
        n162 = case "Channel 2" shown="3" w282 {
          tunnel: ["Part Connected" "Part Connected" w382 "IDLE" "Part Connected"] -> w291
          tunnel: w268 -> [_ _ w381 _ _]
          frame 0, Default {
          }
          frame 1 {
          }
          frame 2 {
            n163 = case shown="False" w381 {
              tunnel: ["Old Part" "Retest"] -> w382
              frame False {
              }
              frame True {
              }
            }
          }
          frame 3 {
            w386 = FALSE
            n164 = property on="CH 2 RES VAL" class="Str"("Value"="") -> ()  [unwired: 2 in, 2 out]
            n165 = property on="CH 2 PASS" class="Bool (strict)"("Value"=w386) -> ()  [unwired: 2 in, 2 out]
            n166 = property on="CH 2 FAIL" class="Bool (strict)"("Value"=w386) -> ()  [unwired: 2 in, 2 out]
          }
          frame 4 {
          }
        }
        n167 = case "Channel 3" shown="2" w281 {
          tunnel: ["Partr Connected" "Part Connected" w372 "IDLE" "Part Connected"] -> w290
          tunnel: w268 -> [_ _ w371 _ _]
          frame 0, Default {
          }
          frame 1 {
          }
          frame 2 {
            n168 = case shown="False" w371 {
              tunnel: ["Old Part" "Retest"] -> w372
              frame False {
              }
              frame True {
              }
            }
          }
          frame 3 {
            w376 = FALSE
            n169 = property on="CH 3 RES VAL" class="Str"("Value"="") -> ()  [unwired: 2 in, 2 out]
            n170 = property on="CH 3 PASS" class="Bool (strict)"("Value"=w376) -> ()  [unwired: 2 in, 2 out]
            n171 = property on="CH 3 FAIL" class="Bool (strict)"("Value"=w376) -> ()  [unwired: 2 in, 2 out]
          }
          frame 4 {
          }
        }
        n172 = case "Channel 4" shown="2" w280 {
          tunnel: ["Part Connected" "Part Connected" w362 "IDLE" "Part Connected"] -> w289
          tunnel: w268 -> [_ _ w361 _ _]
          frame 0, Default {
          }
          frame 1 {
          }
          frame 2 {
            n173 = case shown="False" w361 {
              tunnel: ["Old Part" "Retest"] -> w362
              frame False {
              }
              frame True {
              }
            }
          }
          frame 3 {
            w366 = FALSE
            n174 = property on="CH 4 RES VAL" class="Str"("Value"="") -> ()  [unwired: 2 in, 2 out]
            n175 = property on="CH 4 PASS" class="Bool (strict)"("Value"=w366) -> ()  [unwired: 2 in, 2 out]
            n176 = property on="CH 4 FAIL" class="Bool (strict)"("Value"=w366) -> ()  [unwired: 2 in, 2 out]
          }
          frame 4 {
          }
        }
        n177 = case "Channel 5" shown="2" w267 {
          tunnel: ["Part Connected" "Part Connected" w352 "IDLE" "Part Connected"] -> w288
          tunnel: w268 -> [_ _ w351 _ _]
          frame 0, Default {
          }
          frame 1 {
          }
          frame 2 {
            n178 = case shown="False" w351 {
              tunnel: ["Old Part" "Retest"] -> w352
              frame False {
              }
              frame True {
              }
            }
          }
          frame 3 {
            w356 = FALSE
            n179 = property on="CH 5 RES VAL" class="Str"("Value"="") -> ()  [unwired: 2 in, 2 out]
            n180 = property on="CH 5 PASS" class="Bool (strict)"("Value"=w356) -> ()  [unwired: 2 in, 2 out]
            n181 = property on="CH 5 FAIL" class="Bool (strict)"("Value"=w356) -> ()  [unwired: 2 in, 2 out]
          }
          frame 4 {
          }
        }
        n182 = case "Channel 6" shown="2" w279 {
          tunnel: ["Part Connected" "Part Connected" "Part Connected" w343 "IDLE"] -> w287
          tunnel: w268 -> [_ _ _ w342 _]
          frame 0, Default {
          }
          frame 4 {
          }
          frame 1 {
          }
          frame 2 {
            n183 = case shown="False" w342 {
              tunnel: ["Old Part" "Retest"] -> w343
              frame False {
              }
              frame True {
              }
            }
          }
          frame 3 {
            w347 = FALSE
            n184 = property on="CH 6 RES VAL" class="Str"("Value"="") -> ()  [unwired: 2 in, 2 out]
            n185 = property on="CH 6 PASS" class="Bool (strict)"("Value"=w347) -> ()  [unwired: 2 in, 2 out]
            n186 = property on="CH 6 FAIL" class="Bool (strict)"("Value"=w347) -> ()  [unwired: 2 in, 2 out]
          }
        }
        n187 = case "Channel 7" shown="2" w278 {
          tunnel: ["Part Connected" "Part Connected" w332 "IDLE" "Part Connected"] -> w286
          tunnel: w268 -> [_ _ w331 _ _]
          frame 0, Default {
          }
          frame 1 {
          }
          frame 2 {
            n188 = case shown="True" w331 {
              tunnel: ["Old Part" "Retest"] -> w332
              frame False {
              }
              frame True {
              }
            }
          }
          frame 3 {
            w336 = FALSE
            n189 = property on="CH 7 RES VAL" class="Str"("Value"="") -> ()  [unwired: 2 in, 2 out]
            n190 = property on="CH 7 PASS" class="Bool (strict)"("Value"=w336) -> ()  [unwired: 2 in, 2 out]
            n191 = property on="CH 7 FAIL" class="Bool (strict)"("Value"=w336) -> ()  [unwired: 2 in, 2 out]
          }
          frame 4 {
          }
        }
        n192 = property on="CH 8 STATUS" class="Str"("Value"=w285) -> ()  [unwired: 2 in, 2 out]
        n193 = property on="CH 9 STATUS" class="Str"("Value"=w284) -> ()  [unwired: 2 in, 2 out]
        n194 = property on="CH 10 STATUS" class="Str"("Value"=w283) -> ()  [unwired: 2 in, 2 out]
        n195 = property on="CH1 STATUS" class="Str"("Value"=w292) -> ()  [unwired: 2 in, 2 out]
        n196 = property on="CH 2 STATUS" class="Str"("Value"=w291) -> ()  [unwired: 2 in, 2 out]
        n197 = property on="CH 4 STATUS" class="Str"("Value"=w289) -> ()  [unwired: 2 in, 2 out]
        n198 = property on="CH 5 STATUS" class="Str"("Value"=w288) -> ()  [unwired: 2 in, 2 out]
        n199 = property on="CH 6 STATUS" class="Str"("Value"=w287) -> ()  [unwired: 2 in, 2 out]
        n200 = property on="CH 7 STATUS" class="Str"("Value"=w286) -> ()  [unwired: 2 in, 2 out]
        n201 = property on="CH 3 STATUS" class="Str"("Value"=w290) -> ()  [unwired: 2 in, 2 out]
        n202 = case shown="9" w266 {
          tunnel: [TEST_ENNUM."TIMEOUT" TEST_ENNUM."TIMEOUT" TEST_ENNUM."VALIDATING"] -> w265
          frame 8, Default {
          }
          frame 6 {
            n203 = One Button Dialog(message="NO PART IN REFERENCE CHANNEL", button name ("OK")="OK") -> ()  [unwired: 1 out]
          }
          frame 9 {
          }
        }
      }
      frame "VALIDATING" {
        n204 = Unbundle By Name(w421) -> ("MODE"=w536:string, "RES VALUE 5"=w419:dbl)
        n205 = Equal?(x=w536, y="USER MODE") -> (x = y?=w422:bool)
        n206 = case shown="False" w422 {
          tunnel: [w538 w540] -> w420
          tunnel: w421 -> [w539 w540]
          tunnel: w419 -> [w537 _]
          frame False {
            n207 = Bundle By Name(cluster=w539, "SET VALUE 1"=w537, "SET VALUE 2"=w537, "SET VALUE 3"=w537, "SET VALUE 4"=w537, "SET VALUE 5"=w537, "SET VALUE 6"=w537, "SET VALUE 7"=w537, "SET VALUE 8"=w537, "SET VALUE 9"=w537, "SET VALUE 10"=w537) -> (w538:T1)
          }
          frame True {
          }
        }
        n208 = Unbundle By Name(w420) -> ("PP 1"=w531:i32, "PP 2"=w513:i32, "PP 3"=w512:i32, "PP 4"=w511:i32, "PP 5"=w510:i32, "PP 6"=w509:i32, "PP 7"=w508:i32, "PP 8"=w507:i32, "PP 9"=w506:i32, "PP 10"=w503:i32)
        n209 = Equal?(x=w531, y=2) -> (x = y?=w501:bool)
        n210 = Equal?(x=w531, y=1) -> (x = y?=w500:bool)
        n211 = Equal?(x=w513, y=2) -> (x = y?=w494:bool)
        n212 = Equal?(x=w513, y=1) -> (x = y?=w493:bool)
        n213 = Equal?(x=w512, y=2) -> (x = y?=w492:bool)
        n214 = Equal?(x=w512, y=1) -> (x = y?=w491:bool)
        n215 = Equal?(x=w511, y=2) -> (x = y?=w486:bool)
        n216 = Equal?(x=w511, y=1) -> (x = y?=w487:bool)
        n217 = Equal?(x=w510, y=2) -> (x = y?=w480:bool)
        n218 = Equal?(x=w510, y=1) -> (x = y?=w481:bool)
        n219 = Equal?(x=w509, y=2) -> (x = y?=w477:bool)
        n220 = Equal?(x=w509, y=1) -> (x = y?=w478:bool)
        n221 = Equal?(x=w508, y=2) -> (x = y?=w473:bool)
        n222 = Equal?(x=w508, y=1) -> (x = y?=w472:bool)
        n223 = Equal?(x=w507, y=2) -> (x = y?=w468:bool)
        n224 = Equal?(x=w507, y=1) -> (x = y?=w467:bool)
        n225 = Equal?(x=w506, y=2) -> (x = y?=w463:bool)
        n226 = Equal?(x=w503, y=2) -> (x = y?=w460:bool)
        n227 = Equal?(x=w506, y=1) -> (x = y?=w461:bool)
        n228 = Equal?(x=w503, y=1) -> (x = y?=w462:bool)
        n229 = Or(x=w486, y=w487) -> (x .or. y?=w485:bool)
        n230 = Or(x=w480, y=w481) -> (x .or. y?=w479:bool)
        n231 = Or(x=w477, y=w478) -> (x .or. y?=w476:bool)
        n232 = Or(x=w501, y=w500) -> (x .or. y?=w502:bool)
        n233 = Or(x=w494, y=w493) -> (x .or. y?=w495:bool)
        n234 = Or(x=w492, y=w491) -> (x .or. y?=w490:bool)
        n235 = Or(x=w473, y=w472) -> (x .or. y?=w469:bool)
        n236 = Or(x=w468, y=w467) -> (x .or. y?=w466:bool)
        n237 = Or(x=w463, y=w461) -> (x .or. y?=w459:bool)
        n238 = Or(x=w460, y=w462) -> (x .or. y?=w458:bool)
        n239 = Unbundle By Name(w420) -> ("SET VALUE 1"=w499:dbl, "SET VALUE 2"=w498:dbl, "SET VALUE 3"=w489:dbl, "SET VALUE 4"=w484:dbl, "SET VALUE 5"=w482:dbl, "SET VALUE 6"=w471:dbl, "SET VALUE 7"=w433:dbl, "SET VALUE 8"=w465:dbl, "SET VALUE 9"=w457:dbl, "SET VALUE 10"=w455:dbl, "TOL 1"=w497:dbl, "TOL 2"=w496:dbl, "TOL 3"=w488:dbl, "TOL 4"=w483:dbl, "TOL 5"=w475:dbl, "TOL 6"=w474:dbl, "TOL 7"=w470:dbl, "TOL 8"=w464:dbl, "TOL 9"=w456:dbl, "TOL 10"=w454:dbl, "RES VALUE 1"=w432:dbl, "RES VALUE 2"=w431:dbl, "RES VALUE 3"=w430:dbl, "RES VALUE 4"=w429:dbl, "RES VALUE 5"=w428:dbl, "RES VALUE 6"=w427:dbl, "RES VALUE 7"=w426:dbl, "RES VALUE 8"=w425:dbl, "RES VALUE 9"=w424:dbl, "RES VALUE 10"=w423:dbl)
        n240 = case "Channel 1" shown="True" w502 {
          tunnel: w499 -> [_ w637]
          tunnel: w497 -> [_ w638]
          tunnel: [_ w635] -> w453
          tunnel: [_ w634] -> w452
          tunnel: w432 -> [_ w633]
          tunnel: [_ w632] -> w418
          tunnel: [_ w631] -> w417
          frame False {
          }
          frame True {
            n241 = call "TOL_EQ.vi"("TOL VALUE"=w638, "NOM VALUE"=w637) -> ("MIN"=w631:dbl, "MAX"=w632:dbl)  [unwired: 8 in]
            n242 = In Range and Coerce(upper limit=w632, x=w633, lower limit=w631) -> (In Range?=w636:bool)  [unwired: 1 out]
            n243 = case shown="False" w636 {
              tunnel: [_ TRUE] -> w635
              tunnel: [TRUE _] -> w634
              frame False {
              }
              frame True {
              }
            }
          }
        }
        n244 = case "Channel 2" shown="True" w495 {
          tunnel: w498 -> [_ w627]
          tunnel: w496 -> [_ w628]
          tunnel: [_ w625] -> w451
          tunnel: [_ w624] -> w450
          tunnel: w431 -> [_ w623]
          tunnel: [_ w622] -> w416
          tunnel: [_ w621] -> w415
          frame False {
          }
          frame True {
            n245 = call "TOL_EQ.vi"("TOL VALUE"=w628, "NOM VALUE"=w627) -> ("MIN"=w621:dbl, "MAX"=w622:dbl)  [unwired: 8 in]
            n246 = In Range and Coerce(upper limit=w622, x=w623, lower limit=w621) -> (In Range?=w626:bool)  [unwired: 1 out]
            n247 = case shown="False" w626 {
              tunnel: [_ TRUE] -> w625
              tunnel: [TRUE _] -> w624
              frame False {
              }
              frame True {
              }
            }
          }
        }
        n248 = case "Channel 3" shown="True" w490 {
          tunnel: w489 -> [_ w617]
          tunnel: w488 -> [_ w618]
          tunnel: [_ w615] -> w449
          tunnel: [_ w614] -> w448
          tunnel: w430 -> [_ w613]
          tunnel: [_ w612] -> w414
          tunnel: [_ w611] -> w413
          frame False {
          }
          frame True {
            n249 = call "TOL_EQ.vi"("TOL VALUE"=w618, "NOM VALUE"=w617) -> ("MIN"=w611:dbl, "MAX"=w612:dbl)  [unwired: 8 in]
            n250 = In Range and Coerce(upper limit=w612, x=w613, lower limit=w611) -> (In Range?=w616:bool)  [unwired: 1 out]
            n251 = case shown="True" w616 {
              tunnel: [_ TRUE] -> w615
              tunnel: [TRUE _] -> w614
              frame False {
              }
              frame True {
              }
            }
          }
        }
        n252 = case "Channel 4" shown="True" w485 {
          tunnel: w484 -> [_ w607]
          tunnel: w483 -> [_ w608]
          tunnel: [_ w605] -> w447
          tunnel: [_ w604] -> w446
          tunnel: w429 -> [_ w603]
          tunnel: [_ w602] -> w412
          tunnel: [_ w601] -> w411
          frame False {
          }
          frame True {
            n253 = call "TOL_EQ.vi"("TOL VALUE"=w608, "NOM VALUE"=w607) -> ("MIN"=w601:dbl, "MAX"=w602:dbl)  [unwired: 8 in]
            n254 = In Range and Coerce(upper limit=w602, x=w603, lower limit=w601) -> (In Range?=w606:bool)  [unwired: 1 out]
            n255 = case shown="False" w606 {
              tunnel: [_ TRUE] -> w605
              tunnel: [TRUE _] -> w604
              frame False {
              }
              frame True {
              }
            }
          }
        }
        n256 = case "Channel 5" shown="True" w479 {
          tunnel: w482 -> [_ w597]
          tunnel: w475 -> [_ w598]
          tunnel: [_ w595] -> w445
          tunnel: [_ w594] -> w444
          tunnel: w428 -> [_ w593]
          tunnel: [_ w592] -> w410
          tunnel: [_ w591] -> w409
          frame False {
          }
          frame True {
            n257 = call "TOL_EQ.vi"("TOL VALUE"=w598, "NOM VALUE"=w597) -> ("MIN"=w591:dbl, "MAX"=w592:dbl)  [unwired: 8 in]
            n258 = In Range and Coerce(upper limit=w592, x=w593, lower limit=w591) -> (In Range?=w596:bool)  [unwired: 1 out]
            n259 = case shown="False" w596 {
              tunnel: [_ TRUE] -> w595
              tunnel: [TRUE _] -> w594
              frame False {
              }
              frame True {
              }
            }
          }
        }
        n260 = case "Channel 6" shown="False" w476 {
          tunnel: w471 -> [_ w587]
          tunnel: w474 -> [_ w588]
          tunnel: [_ w585] -> w443
          tunnel: [_ w584] -> w442
          tunnel: w427 -> [_ w583]
          tunnel: [_ w582] -> w408
          tunnel: [_ w581] -> w407
          frame False {
          }
          frame True {
            n261 = call "TOL_EQ.vi"("TOL VALUE"=w588, "NOM VALUE"=w587) -> ("MIN"=w581:dbl, "MAX"=w582:dbl)  [unwired: 8 in]
            n262 = In Range and Coerce(upper limit=w582, x=w583, lower limit=w581) -> (In Range?=w586:bool)  [unwired: 1 out]
            n263 = case shown="False" w586 {
              tunnel: [_ TRUE] -> w585
              tunnel: [TRUE _] -> w584
              frame False {
              }
              frame True {
              }
            }
          }
        }
        n264 = case "Channel 10" shown="False" w458 {
          tunnel: w455 -> [_ w547]
          tunnel: w454 -> [_ w548]
          tunnel: [_ w545] -> w435
          tunnel: [_ w544] -> w434
          tunnel: w423 -> [_ w543]
          tunnel: [_ w542] -> w400
          tunnel: [_ w541] -> w399
          frame False {
          }
          frame True {
            n265 = call "TOL_EQ.vi"("TOL VALUE"=w548, "NOM VALUE"=w547) -> ("MIN"=w541:dbl, "MAX"=w542:dbl)  [unwired: 8 in]
            n266 = In Range and Coerce(upper limit=w542, x=w543, lower limit=w541) -> (In Range?=w546:bool)  [unwired: 1 out]
            n267 = case shown="False" w546 {
              tunnel: [_ TRUE] -> w545
              tunnel: [TRUE _] -> w544
              frame False {
              }
              frame True {
              }
            }
          }
        }
        n268 = case "Channel 7" shown="False" w469 {
          tunnel: w470 -> [_ w578]
          tunnel: [_ w576] -> w441
          tunnel: [_ w575] -> w440
          tunnel: w433 -> [_ w574]
          tunnel: w426 -> [_ w573]
          tunnel: [_ w572] -> w406
          tunnel: [_ w571] -> w405
          frame False {
          }
          frame True {
            n269 = call "TOL_EQ.vi"("TOL VALUE"=w578, "NOM VALUE"=w574) -> ("MIN"=w571:dbl, "MAX"=w572:dbl)  [unwired: 8 in]
            n270 = In Range and Coerce(upper limit=w572, x=w573, lower limit=w571) -> (In Range?=w577:bool)  [unwired: 1 out]
            n271 = case shown="False" w577 {
              tunnel: [_ TRUE] -> w576
              tunnel: [TRUE _] -> w575
              frame False {
              }
              frame True {
              }
            }
          }
        }
        n272 = case "Channel 8" shown="True" w466 {
          tunnel: w465 -> [_ w567]
          tunnel: w464 -> [_ w568]
          tunnel: [_ w565] -> w439
          tunnel: [_ w564] -> w438
          tunnel: w425 -> [_ w563]
          tunnel: [_ w562] -> w404
          tunnel: [_ w561] -> w403
          frame False {
          }
          frame True {
            n273 = call "TOL_EQ.vi"("TOL VALUE"=w568, "NOM VALUE"=w567) -> ("MIN"=w561:dbl, "MAX"=w562:dbl)  [unwired: 8 in]
            n274 = In Range and Coerce(upper limit=w562, x=w563, lower limit=w561) -> (In Range?=w566:bool)  [unwired: 1 out]
            n275 = case shown="False" w566 {
              tunnel: [_ TRUE] -> w565
              tunnel: [TRUE _] -> w564
              frame False {
              }
              frame True {
              }
            }
          }
        }
        n276 = case "Channel 9" shown="False" w459 {
          tunnel: w457 -> [_ w557]
          tunnel: w456 -> [_ w558]
          tunnel: [_ w555] -> w437
          tunnel: [_ w554] -> w436
          tunnel: w424 -> [_ w553]
          tunnel: [_ w552] -> w402
          tunnel: [_ w551] -> w401
          frame False {
          }
          frame True {
            n277 = call "TOL_EQ.vi"("TOL VALUE"=w558, "NOM VALUE"=w557) -> ("MIN"=w551:dbl, "MAX"=w552:dbl)  [unwired: 8 in]
            n278 = In Range and Coerce(upper limit=w552, x=w553, lower limit=w551) -> (In Range?=w556:bool)  [unwired: 1 out]
            n279 = case shown="False" w556 {
              tunnel: [_ TRUE] -> w555
              tunnel: [TRUE _] -> w554
              frame False {
              }
              frame True {
              }
            }
          }
        }
        n280 = Bundle By Name(cluster=w420, "CH  PASS  1"=w453, "CH  PASS 2"=w451, "CH  PASS 3"=w449, "CH  PASS 4"=w447, "CH  PASS 5"=w445, "CH  PASS 6"=w443, "CH  PASS 7"=w441, "CH  PASS 8"=w439, "CH  PASS 9"=w437, "CH  PASS 10"=w435, "CH  FAIL 1"=w452, "CH  FAIL 2"=w450, "CH  FAIL 3"=w448, "CH  FAIL 4"=w446, "CH  FAIL 5"=w444, "CH  FAIL 6"=w442, "CH  FAIL 7"=w440, "CH  FAIL 8"=w438, "CH  FAIL 9"=w436, "CH  FAIL 10"=w434, "CH1 MIN TOL"=w417, "CH2 MIN TOL"=w415, "CH3 MIN TOL"=w413, "CH4 MIN TOL"=w411, "CH5 MIN TOL"=w409, "CH6 MIN TOL"=w407, "CH7 MIN TOL"=w405, "CH8 MIN TOL"=w403, "CH9 MIN TOL"=w401, "CH10 MIN TOL"=w399, "CH1 MAX TOL"=w418, "CH2 MAX TOL"=w416, "CH3 MAX TOL"=w414, "CH4 MAX TOL"=w412, "CH5 MAX TOL"=w410, "CH6 MAX TOL"=w408, "CH7 MAX TOL"=w406, "CH8 MAX TOL"=w404, "CH9 MAX TOL"=w402, "CH10 MAX TOL"=w400) -> (w534:T1)
      }
      frame "RESULT" {
        n281 = Unbundle By Name(w641) -> ("PP 1"=w677:i32, "PP 2"=w674:i32, "PP 3"=w671:i32, "PP 4"=w668:i32, "PP 5"=w665:i32, "PP 6"=w662:i32, "PP 7"=w659:i32, "PP 8"=w656:i32, "PP 9"=w653:i32, "PP 10"=w650:i32, "CH  PASS  1"=w676:bool, "CH  PASS 2"=w673:bool, "CH  PASS 3"=w670:bool, "CH  PASS 4"=w667:bool, "CH  PASS 5"=w664:bool, "CH  PASS 6"=w661:bool, "CH  PASS 7"=w658:bool, "CH  PASS 8"=w655:bool, "CH  PASS 9"=w652:bool, "CH  PASS 10"=w649:bool, "CH  FAIL 1"=w675:bool, "CH  FAIL 2"=w672:bool, "CH  FAIL 3"=w669:bool, "CH  FAIL 4"=w666:bool, "CH  FAIL 5"=w663:bool, "CH  FAIL 6"=w660:bool, "CH  FAIL 7"=w657:bool, "CH  FAIL 8"=w654:bool, "CH  FAIL 9"=w651:bool, "CH  FAIL 10"=w648:bool, "RES VALUE 1"=w644:dbl, "RES VALUE 2"=w702:dbl, "RES VALUE 3"=w701:dbl, "RES VALUE 4"=w700:dbl, "RES VALUE 5"=w699:dbl, "RES VALUE 6"=w698:dbl, "RES VALUE 7"=w647:dbl, "RES VALUE 8"=w697:dbl, "RES VALUE 9"=w696:dbl, "RES VALUE 10"=w695:dbl, "PP 1"=w645:i32, "PP 2"=w685:i32, "PP 3"=w684:i32, "PP 4"=w683:i32, "PP 5"=w682:i32, "PP 6"=w681:i32, "PP 7"=w646:i32, "PP 8"=w680:i32, "PP 9"=w679:i32, "PP 10"=w678:i32)
        n282 = case shown="2" w677 {
          tunnel: w676 -> [_ w750 w752]
          tunnel: w675 -> [_ w749 w751]
          frame 0, Default {
          }
          frame 1 {
            n283 = property on="CH 1 PASS" class="Bool (strict)"("Value"=w750) -> ()  [unwired: 2 in, 2 out]
            n284 = property on="CH 1 FAIL" class="Bool (strict)"("Value"=w749) -> ()  [unwired: 2 in, 2 out]
          }
          frame 2 {
            n285 = property on="CH 1 FAIL" class="Bool (strict)"("Value"=w751) -> ()  [unwired: 2 in, 2 out]
            n286 = property on="CH 1 PASS" class="Bool (strict)"("Value"=w752) -> ()  [unwired: 2 in, 2 out]
          }
        }
        n287 = case shown="3" w645 {
          tunnel: w644 -> [_ w705 w709 _]
          tunnel: ["0" w704 w708 ""] -> w643
          frame 0, Default {
          }
          frame 1 {
            n288 = Number To Fractional String(use system decimal point (T)=TRUE, number=w705, precision (6)=i16 3) -> (F-format string=w704:string)  [unwired: 1 in]
          }
          frame 2 {
            n289 = Number To Fractional String(use system decimal point (T)=TRUE, number=w709, precision (6)=i16 3) -> (F-format string=w708:string)  [unwired: 1 in]
          }
          frame 3 {
          }
        }
        n290 = case shown="3" w685 {
          tunnel: w702 -> [_ w834 w838 _]
          tunnel: ["0" w833 w837 ""] -> w694
          frame 0, Default {
          }
          frame 1 {
            n291 = Number To Fractional String(use system decimal point (T)=TRUE, number=w834, precision (6)=i16 3) -> (F-format string=w833:string)  [unwired: 1 in]
          }
          frame 2 {
            n292 = Number To Fractional String(use system decimal point (T)=TRUE, number=w838, precision (6)=i16 3) -> (F-format string=w837:string)  [unwired: 1 in]
          }
          frame 3 {
          }
        }
        n293 = case shown="0, Default" w684 {
          tunnel: w701 -> [_ w825 w829 _]
          tunnel: ["" w824 w828 _] -> w693
          frame 0, Default {
          }
          frame 1 {
            n294 = Number To Fractional String(use system decimal point (T)=TRUE, number=w825, precision (6)=i16 3) -> (F-format string=w824:string)  [unwired: 1 in]
          }
          frame 2 {
            n295 = Number To Fractional String(use system decimal point (T)=TRUE, number=w829, precision (6)=i16 3) -> (F-format string=w828:string)  [unwired: 1 in]
          }
          frame 3 {
          }
        }
        n296 = case shown="1" w683 {
          tunnel: w700 -> [_ w815 w819 _]
          tunnel: ["0" w814 w818 ""] -> w692
          frame 0, Default {
          }
          frame 1 {
            n297 = Number To Fractional String(use system decimal point (T)=TRUE, number=w815, precision (6)=i16 3) -> (F-format string=w814:string)  [unwired: 1 in]
          }
          frame 2 {
            n298 = Number To Fractional String(use system decimal point (T)=TRUE, number=w819, precision (6)=i16 3) -> (F-format string=w818:string)  [unwired: 1 in]
          }
          frame 3 {
          }
        }
        n299 = case shown="2" w682 {
          tunnel: w699 -> [_ w805 w808 _]
          tunnel: ["0" w804 w809 ""] -> w691
          frame 0, Default {
          }
          frame 1 {
            n300 = Number To Fractional String(use system decimal point (T)=TRUE, number=w805, precision (6)=i16 3) -> (F-format string=w804:string)  [unwired: 1 in]
          }
          frame 2 {
            n301 = Number To Fractional String(use system decimal point (T)=TRUE, number=w808, precision (6)=i16 3) -> (F-format string=w809:string)  [unwired: 1 in]
          }
          frame 3 {
          }
        }
        n302 = case shown="3" w681 {
          tunnel: w698 -> [_ w795 w799 _]
          tunnel: ["0" w794 w798 ""] -> w690
          frame 0, Default {
          }
          frame 1 {
            n303 = Number To Fractional String(use system decimal point (T)=TRUE, number=w795, precision (6)=i16 3) -> (F-format string=w794:string)  [unwired: 1 in]
          }
          frame 2 {
            n304 = Number To Fractional String(use system decimal point (T)=TRUE, number=w799, precision (6)=i16 3) -> (F-format string=w798:string)  [unwired: 1 in]
          }
          frame 3 {
          }
        }
        n305 = case shown="3" w646 {
          tunnel: w647 -> [_ w785 w789 _]
          tunnel: ["0" w784 w788 ""] -> w689
          frame 0, Default {
          }
          frame 1 {
            n306 = Number To Fractional String(use system decimal point (T)=TRUE, number=w785, precision (6)=i16 3) -> (F-format string=w784:string)  [unwired: 1 in]
          }
          frame 2 {
            n307 = Number To Fractional String(use system decimal point (T)=TRUE, number=w789, precision (6)=i16 3) -> (F-format string=w788:string)  [unwired: 1 in]
          }
          frame 3 {
          }
        }
        n308 = case shown="3" w680 {
          tunnel: w697 -> [_ w775 w779 _]
          tunnel: ["0" w774 w778 ""] -> w688
          frame 0, Default {
          }
          frame 1 {
            n309 = Number To Fractional String(use system decimal point (T)=TRUE, number=w775, precision (6)=i16 3) -> (F-format string=w774:string)  [unwired: 1 in]
          }
          frame 2 {
            n310 = Number To Fractional String(use system decimal point (T)=TRUE, number=w779, precision (6)=i16 3) -> (F-format string=w778:string)  [unwired: 1 in]
          }
          frame 3 {
          }
        }
        n311 = case shown="3" w679 {
          tunnel: w696 -> [_ w765 w769 _]
          tunnel: ["" w764 w768 ""] -> w687
          frame 0, Default {
          }
          frame 1 {
            n312 = Number To Fractional String(use system decimal point (T)=TRUE, number=w765, precision (6)=i16 3) -> (F-format string=w764:string)  [unwired: 1 in]
          }
          frame 2 {
            n313 = Number To Fractional String(use system decimal point (T)=TRUE, number=w769, precision (6)=i16 3) -> (F-format string=w768:string)  [unwired: 1 in]
          }
          frame 3 {
          }
        }
        n314 = case shown="3" w678 {
          tunnel: w695 -> [_ w757 w759 _]
          tunnel: ["0" w756 w758 ""] -> w686
          frame 0, Default {
          }
          frame 1 {
            n315 = Number To Fractional String(use system decimal point (T)=TRUE, number=w757, precision (6)=i16 3) -> (F-format string=w756:string)  [unwired: 1 in]
          }
          frame 2 {
            n316 = Number To Fractional String(use system decimal point (T)=TRUE, number=w759, precision (6)=i16 3) -> (F-format string=w758:string)  [unwired: 1 in]
          }
          frame 3 {
          }
        }
        n317 = property on="CH 1 RES VAL" class="Str"("Value"=w643) -> ()  [unwired: 2 in, 2 out]
        n318 = property on="CH 2 RES VAL" class="Str"("Value"=w694) -> ()  [unwired: 2 in, 2 out]
        n319 = property on="CH 3 RES VAL" class="Str"("Value"=w693) -> ()  [unwired: 2 in, 2 out]
        n320 = property on="CH 4 RES VAL" class="Str"("Value"=w692) -> ()  [unwired: 2 in, 2 out]
        n321 = property on="CH 5 RES VAL" class="Str"("Value"=w691) -> ()  [unwired: 2 in, 2 out]
        n322 = property on="CH 6 RES VAL" class="Str"("Value"=w690) -> ()  [unwired: 2 in, 2 out]
        n323 = property on="CH 7 RES VAL" class="Str"("Value"=w689) -> ()  [unwired: 2 in, 2 out]
        n324 = property on="CH 8 RES VAL" class="Str"("Value"=w688) -> ()  [unwired: 2 in, 2 out]
        n325 = property on="CH 9 RES VAL" class="Str"("Value"=w687) -> ()  [unwired: 2 in, 2 out]
        n326 = property on="CH 10 RES VAL" class="Str"("Value"=w686) -> ()  [unwired: 2 in, 2 out]
        n327 = case shown="2" w674 {
          tunnel: w673 -> [_ w746 w748 _]
          tunnel: w672 -> [_ w745 w747 _]
          frame 0, Default {
          }
          frame 1 {
            n328 = property on="CH 2 PASS" class="Bool (strict)"("Value"=w746) -> ()  [unwired: 2 in, 2 out]
            n329 = property on="CH 2 FAIL" class="Bool (strict)"("Value"=w745) -> ()  [unwired: 2 in, 2 out]
          }
          frame 2 {
            n330 = property on="CH 2 PASS" class="Bool (strict)"("Value"=w748) -> ()  [unwired: 2 in, 2 out]
            n331 = property on="CH 2 FAIL" class="Bool (strict)"("Value"=w747) -> ()  [unwired: 2 in, 2 out]
          }
          frame 3 {
          }
        }
        n332 = case shown="1" w671 {
          tunnel: w670 -> [_ w742 w744 _]
          tunnel: w669 -> [_ w741 w743 _]
          frame 0, Default {
          }
          frame 1 {
            n333 = property on="CH 3 PASS" class="Bool (strict)"("Value"=w742) -> ()  [unwired: 2 in, 2 out]
            n334 = property on="CH 3 FAIL" class="Bool (strict)"("Value"=w741) -> ()  [unwired: 2 in, 2 out]
          }
          frame 2 {
            n335 = property on="CH 3 PASS" class="Bool (strict)"("Value"=w744) -> ()  [unwired: 2 in, 2 out]
            n336 = property on="CH 3 FAIL" class="Bool (strict)"("Value"=w743) -> ()  [unwired: 2 in, 2 out]
          }
          frame 3 {
          }
        }
        n337 = case shown="1" w668 {
          tunnel: w667 -> [_ w738 w740 _]
          tunnel: w666 -> [_ w737 w739 _]
          frame 0, Default {
          }
          frame 1 {
            n338 = property on="CH 4 PASS" class="Bool (strict)"("Value"=w738) -> ()  [unwired: 2 in, 2 out]
            n339 = property on="CH 4 FAIL" class="Bool (strict)"("Value"=w737) -> ()  [unwired: 2 in, 2 out]
          }
          frame 2 {
            n340 = property on="CH 4 PASS" class="Bool (strict)"("Value"=w740) -> ()  [unwired: 2 in, 2 out]
            n341 = property on="CH 4 FAIL" class="Bool (strict)"("Value"=w739) -> ()  [unwired: 2 in, 2 out]
          }
          frame 3 {
          }
        }
        n342 = case shown="1" w665 {
          tunnel: w664 -> [_ w734 w736 _]
          tunnel: w663 -> [_ w733 w735 _]
          frame 0, Default {
          }
          frame 1 {
            n343 = property on="CH 5 PASS" class="Bool (strict)"("Value"=w734) -> ()  [unwired: 2 in, 2 out]
            n344 = property on="CH 5 FAIL" class="Bool (strict)"("Value"=w733) -> ()  [unwired: 2 in, 2 out]
          }
          frame 2 {
            n345 = property on="CH 5 PASS" class="Bool (strict)"("Value"=w736) -> ()  [unwired: 2 in, 2 out]
            n346 = property on="CH 5 FAIL" class="Bool (strict)"("Value"=w735) -> ()  [unwired: 2 in, 2 out]
          }
          frame 3 {
          }
        }
        n347 = case shown="1" w662 {
          tunnel: w661 -> [_ w730 w732 _]
          tunnel: w660 -> [_ w729 w731 _]
          frame 0, Default {
          }
          frame 1 {
            n348 = property on="CH 6 PASS" class="Bool (strict)"("Value"=w730) -> ()  [unwired: 2 in, 2 out]
            n349 = property on="CH 6 FAIL" class="Bool (strict)"("Value"=w729) -> ()  [unwired: 2 in, 2 out]
          }
          frame 2 {
            n350 = property on="CH 6 FAIL" class="Bool (strict)"("Value"=w731) -> ()  [unwired: 2 in, 2 out]
            n351 = property on="CH 6 PASS" class="Bool (strict)"("Value"=w732) -> ()  [unwired: 2 in, 2 out]
          }
          frame 3 {
          }
        }
        n352 = case shown="1" w659 {
          tunnel: w658 -> [_ w726 w728 _]
          tunnel: w657 -> [_ w725 w727 _]
          frame 0, Default {
          }
          frame 1 {
            n353 = property on="CH 7 PASS" class="Bool (strict)"("Value"=w726) -> ()  [unwired: 2 in, 2 out]
            n354 = property on="CH 7 FAIL" class="Bool (strict)"("Value"=w725) -> ()  [unwired: 2 in, 2 out]
          }
          frame 2 {
            n355 = property on="CH 7 PASS" class="Bool (strict)"("Value"=w728) -> ()  [unwired: 2 in, 2 out]
            n356 = property on="CH 7 FAIL" class="Bool (strict)"("Value"=w727) -> ()  [unwired: 2 in, 2 out]
          }
          frame 3 {
          }
        }
        n357 = case shown="1" w656 {
          tunnel: w655 -> [_ w722 w724 _]
          tunnel: w654 -> [_ w721 w723 _]
          frame 0, Default {
          }
          frame 1 {
            n358 = property on="CH 8 PASS" class="Bool (strict)"("Value"=w722) -> ()  [unwired: 2 in, 2 out]
            n359 = property on="CH 8 FAIL" class="Bool (strict)"("Value"=w721) -> ()  [unwired: 2 in, 2 out]
          }
          frame 2 {
            n360 = property on="CH 8 PASS" class="Bool (strict)"("Value"=w724) -> ()  [unwired: 2 in, 2 out]
            n361 = property on="CH 8 FAIL" class="Bool (strict)"("Value"=w723) -> ()  [unwired: 2 in, 2 out]
          }
          frame 3 {
          }
        }
        n362 = case shown="1" w653 {
          tunnel: w652 -> [_ w718 w720 _]
          tunnel: w651 -> [_ w717 w719 _]
          frame 0, Default {
          }
          frame 1 {
            n363 = property on="CH 9 PASS" class="Bool (strict)"("Value"=w718) -> ()  [unwired: 2 in, 2 out]
            n364 = property on="CH 9 FAIL" class="Bool (strict)"("Value"=w717) -> ()  [unwired: 2 in, 2 out]
          }
          frame 2 {
            n365 = property on="CH 9 PASS" class="Bool (strict)"("Value"=w720) -> ()  [unwired: 2 in, 2 out]
            n366 = property on="CH 9 FAIL" class="Bool (strict)"("Value"=w719) -> ()  [unwired: 2 in, 2 out]
          }
          frame 3 {
          }
        }
        n367 = case shown="1" w650 {
          tunnel: w649 -> [_ w714 w716 _]
          tunnel: w648 -> [_ w713 w715 _]
          frame 0, Default {
          }
          frame 1 {
            n368 = property on="CH 10  PASS" class="Bool (strict)"("Value"=w714) -> ()  [unwired: 2 in, 2 out]
            n369 = property on="CH 10 FAIL" class="Bool (strict)"("Value"=w713) -> ()  [unwired: 2 in, 2 out]
          }
          frame 2 {
            n370 = property on="CH 10  PASS" class="Bool (strict)"("Value"=w716) -> ()  [unwired: 2 in, 2 out]
            n371 = property on="CH 10 FAIL" class="Bool (strict)"("Value"=w715) -> ()  [unwired: 2 in, 2 out]
          }
          frame 3 {
          }
        }
      }
      frame "LED_SEQ" {
        w857 = u16 10 items=["1.0"=10, "1.5"=15, "2.0"=20] ("stop bits (10: 1 bit)")
        w842 = 0.0 ("element")
        # "CHANNEL 9"
        # "CHANNEL 8"
        # "CHANNEL 7"
        # "CHANNEL 6"
        # "CHANNEL 5"
        # "CHANNEL 4"
        # "CHANNEL 3"
        # "CHANNEL 2"
        # "CHANNEL 1"
        n372 = Unbundle By Name(w860) -> ("VISA resource name"=w861:refnum<visa-resource-name>, "PP 1"=w890:i32, "PP 2"=w888:i32, "PP 3"=w886:i32, "PP 4"=w884:i32, "PP 5"=w882:i32, "PP 6"=w880:i32, "PP 7"=w878:i32, "PP 8"=w876:i32, "PP 9"=w874:i32, "PP 10"=w872:i32, "CH  PASS  1"=w889:bool, "CH  PASS 2"=w887:bool, "CH  PASS 3"=w885:bool, "CH  PASS 4"=w883:bool, "CH  PASS 5"=w881:bool, "CH  PASS 6"=w879:bool, "CH  PASS 7"=w877:bool, "CH  PASS 8"=w875:bool, "CH  PASS 9"=w873:bool, "CH  PASS 10"=w871:bool)
        n373 = case shown="1" w890 {
          tunnel: w889 -> [_ w1002 w1009 _]
          tunnel: [0.0 ("t") w1003 w1006 0.0 ("f")] -> w870
          frame 0, Default {
          }
          frame 1 {
            n374 = Select(t=4.0, s=w1002, f=5.0) -> (s? t:f=w1003:dbl)
          }
          frame 2 {
            n375 = Select(t=4.0, s=w1009, f=5.0) -> (s? t:f=w1006:dbl)
          }
          frame 3 {
          }
        }
        n376 = case shown="0, Default" w888 {
          tunnel: w887 -> [_ w993 w999 _]
          tunnel: [0.0 ("t") w992 w996 0.0 ("f")] -> w869
          frame 0, Default {
          }
          frame 1 {
            n377 = Select(t=4.0, s=w993, f=5.0) -> (s? t:f=w992:dbl)
          }
          frame 2 {
            n378 = Select(t=4.0, s=w999, f=5.0) -> (s? t:f=w996:dbl)
          }
          frame 3 {
          }
        }
        n379 = case shown="0, Default" w886 {
          tunnel: w885 -> [_ w982 w989 _]
          tunnel: [0.0 ("t") w983 w986 0.0 ("f")] -> w868
          frame 0, Default {
          }
          frame 1 {
            n380 = Select(t=4.0, s=w982, f=5.0) -> (s? t:f=w983:dbl)
          }
          frame 2 {
            n381 = Select(t=4.0, s=w989, f=5.0) -> (s? t:f=w986:dbl)
          }
          frame 3 {
          }
        }
        n382 = case shown="0, Default" w884 {
          tunnel: w883 -> [_ w973 w979 _]
          tunnel: [0.0 ("t") w972 w976 0.0 ("f")] -> w867
          frame 0, Default {
          }
          frame 1 {
            n383 = Select(t=4.0, s=w973, f=5.0) -> (s? t:f=w972:dbl)
          }
          frame 2 {
            n384 = Select(t=4.0, s=w979, f=5.0) -> (s? t:f=w976:dbl)
          }
          frame 3 {
          }
        }
        n385 = case shown="0, Default" w882 {
          tunnel: w881 -> [_ w963 w969 _]
          tunnel: [0.0 ("t") w962 w966 0.0 ("f")] -> w866
          frame 0, Default {
          }
          frame 1 {
            n386 = Select(t=4.0, s=w963, f=5.0) -> (s? t:f=w962:dbl)
          }
          frame 2 {
            n387 = Select(t=4.0, s=w969, f=5.0) -> (s? t:f=w966:dbl)
          }
          frame 3 {
          }
        }
        n388 = case shown="0, Default" w880 {
          tunnel: w879 -> [_ w953 w959 _]
          tunnel: [0.0 ("t") w952 w956 0.0 ("f")] -> w865
          frame 0, Default {
          }
          frame 1 {
            n389 = Select(t=4.0, s=w953, f=5.0) -> (s? t:f=w952:dbl)
          }
          frame 2 {
            n390 = Select(t=4.0, s=w959, f=5.0) -> (s? t:f=w956:dbl)
          }
          frame 3 {
          }
        }
        n391 = case shown="0, Default" w878 {
          tunnel: w877 -> [_ w943 w949 _]
          tunnel: [0.0 ("t") w942 w946 0.0 ("f")] -> w864
          frame 0, Default {
          }
          frame 1 {
            n392 = Select(t=4.0, s=w943, f=5.0) -> (s? t:f=w942:dbl)
          }
          frame 2 {
            n393 = Select(t=4.0, s=w949, f=5.0) -> (s? t:f=w946:dbl)
          }
          frame 3 {
          }
        }
        n394 = case shown="0, Default" w876 {
          tunnel: w875 -> [_ w933 w939 _]
          tunnel: [0.0 ("t") w932 w936 0.0 ("f")] -> w863
          frame 0, Default {
          }
          frame 1 {
            n395 = Select(t=4.0, s=w933, f=5.0) -> (s? t:f=w932:dbl)
          }
          frame 2 {
            n396 = Select(t=4.0, s=w939, f=5.0) -> (s? t:f=w936:dbl)
          }
          frame 3 {
          }
        }
        n397 = case shown="0, Default" w874 {
          tunnel: w873 -> [_ w923 w929 _]
          tunnel: [0.0 ("t") w922 w926 0.0 ("f")] -> w862
          frame 0, Default {
          }
          frame 1 {
            n398 = Select(t=4.0, s=w923, f=5.0) -> (s? t:f=w922:dbl)
          }
          frame 2 {
            n399 = Select(t=4.0, s=w929, f=5.0) -> (s? t:f=w926:dbl)
          }
          frame 3 {
          }
        }
        n400 = case shown="0, Default" w872 {
          tunnel: w871 -> [_ w913 w919 _]
          tunnel: [0.0 ("t") w912 w916 0.0 ("f")] -> w853
          frame 0, Default {
          }
          frame 1 {
            n401 = Select(t=4.0, s=w913, f=5.0) -> (s? t:f=w912:dbl)
          }
          frame 2 {
            n402 = Select(t=4.0, s=w919, f=5.0) -> (s? t:f=w916:dbl)
          }
          frame 3 {
          }
        }
        n403 = call ".INI READ.vi"() -> ("MODE"=w848:string, "TEST MODE"=w851:string, "TIME"=w843:dbl)  [unwired: 4 in, 5 out]
        n404 = Equal?(x=w851, y="RETEST") -> (x = y?=w849:bool)
        n405 = case shown="False" w849 {
          tunnel: [1.0 ("element") 2.0 ("element")] -> w845
          frame False {
          }
          frame True {
          }
        }
        n406 = Equal?(x=w848, y="CHANNEL REF MODE") -> (x = y?=w846:bool)
        n407 = case shown="False" w846 {
          tunnel: [1.0 ("element") 2.0 ("element")] -> w844
          frame False {
          }
          frame True {
          }
        }
        n408 = Build Array(w842, w842, w842, w842, w842, w842, w845, w844, w842, w843, w842, w842, w842, w842, w842, w842, w842, w842, w842, w842, w842, w842, w842, w842, w842, w842, w842, w842, w842, w842, w842, w842, w842, w842, w842, w842, w842, w842, w842, w842, w870, w869, w868, w867, w866, w865, w864, w863, w862, w853, 0.0 ("element"), 187.0 ("element")) -> (w859:dbl[])
        n409 = flat-sequence {
          tunnel: w859 -> [w910]
          tunnel: [w910] -> w852
          frame #0 {
            n410 = Wait (ms)(milliseconds to wait=u32 0) -> ()  [unwired: 1 out]
          }
        }
        n411 = call-poly "VISA Configure Serial Port"("VISA resource name"=w861, "timeout (10sec)"=u32 2000, "baud rate (9600)"=u32 115200, "data bits (8)"=u16 8, "parity (0:none)"=enum16{"None", "Odd", "Even", "Mark", "Space"}."None", "stop bits (10: 1 bit)"=w857) -> ("VISA resource name out"=w902:refnum<visa-resource-name>, "error out"=w901:errorcluster)  [unwired: 8 in]
        n412 = VISA Open(timeout (0)=u32 2000 ("VISA Open timeout (0)"), error in (no error)=w901, VISA resource name=w902) -> (VISA resource name=w893:refnum<visa-resource-name>, error out=w894:errorcluster)  [unwired: 2 in]
        n413 = flat-sequence {
          tunnel: [w1013] -> w895
          tunnel: w894 -> [w1013]
          tunnel: w893 -> [w1012]
          tunnel: [w1012] -> w892
          frame #0 {
            n414 = Wait (ms)(milliseconds to wait=u32 0) -> ()  [unwired: 1 out]
          }
        }
        n415 = Byte Array To String(unsigned byte array=w852) -> (string=w854:string)
        n416 = VISA Write(VISA resource name=w892, write buffer=w854, error in (no error)=w895) -> (VISA resource name out=w897:refnum<visa-resource-name>, error out=w896:errorcluster)  [unwired: 1 out]
        n417 = VISA Close(VISA resource name=w897, error in (no error)=w896) -> (error out=w858:errorcluster)
      }
      frame "READY TO PRINT" {
        n418 = Unbundle By Name(w1021) -> ("RES VALUE 1"=w1018:dbl)
        n419 = call "Label Generation.vi"() -> ("error out 2"=w1016:errorcluster)  [unwired: 7 in, 4 out]
        n420 = Number To Decimal String(number=w1018) -> (decimal integer string=w1020:string)  [unwired: 1 in]
        n421 = case shown="No Error" w1016 {
          frame No Error {
            n422 = property on="Printer" class="Bool (strict)"("Colors [4]"=cluster{u32, u32}[] [{1244968, 65309}]) -> ()  [unwired: 2 in, 2 out]
          }
          frame Error {
            n423 = property on="Printer" class="Bool (strict)"("Colors [4]"=cluster{u32, u32}[] [{16720896, 16731178}]) -> ()  [unwired: 2 in, 2 out]
          }
        }
        n424 = call <userlib>:"String to 1D Array__ogtk.vi"("string"=w1020) -> ("Array of Strings"=w1019:string[])  [unwired: 10 in]
        n425 = call "Update Serial Number1.vi"() -> ("Serial number"=w1014:string)  [unwired: 9 in, 2 out]
        n426 = call "Label Generation.vi"("Resistance Value"=w1019, "Serial No"=w1014) -> ("Printer Command"=→"Printer Command":string)  [unwired: 5 in, 4 out]
      }
      frame "REPORT " {
        n427 = call ".INI READ.vi"() -> ("MODE"=w1025:string, "TEST MODE"=w1026:string)  [unwired: 4 in, 6 out]
        n428 = call "Report Gen Title_Folder.vi"() -> ()  [unwired: 12 in]
        n429 = Equal?(x=w1026, y="RETEST") -> (x = y?=w1028:bool)
        n430 = Select(t=TRUE, s=w1028, f=FALSE) -> (s? t:f=w1027:bool)
        n431 = stacked-sequence {
          tunnel: w1032 -> [w1038 w1117 w1196 w1275 w1354 w1433 w1512 w1591 w1670 w1749]
          tunnel: w1027 -> [w1037 w1116 w1195 w1274 w1353 w1432 w1511 w1590 w1669 w1748]
          tunnel: w1027 -> [w1036 w1114 w1193 w1272 w1351 w1430 w1509 w1588 w1667 w1746]
          tunnel: w1025 -> [w1035 w1115 w1194 w1273 w1352 w1431 w1510 w1589 w1668 w1747]
          tunnel: "appended path" -> [w1034 w1113 w1192 w1271 w1350 w1429 w1508 w1587 w1666 w1745]
          frame #0 {
            # "Channel 1 data log"
            n432 = Unbundle By Name(w1038) -> ("PP 1"=w1039:i32)
            n433 = case shown="1" w1039 {
              tunnel: w1038 -> [_ w1049 w1075]
              tunnel: w1034 -> [_ w1050 w1078]
              tunnel: w1037 -> [_ w1042 w1077]
              tunnel: w1036 -> [_ _ w1076]
              tunnel: w1035 -> [_ w1041 w1074]
              frame 0, Default {
              }
              frame 1 {
                n434 = Unbundle By Name(w1049) -> ("SET VALUE 1"=w1069:dbl, "TOL 1"=w1067:dbl, "RES VALUE 1"=w1065:dbl, "CH  PASS  1"=w1063:bool, "CH1 MAX TOL"=w1048:dbl, "CH1 MIN TOL"=w1046:dbl)
                n435 = case shown="True" w1063 {
                  tunnel: ["FAIL" "PASS"] -> w1056
                  frame False {
                  }
                  frame True {
                  }
                }
                n436 = case shown="True" w1042 {
                  tunnel: ["NORMAL" "RETEST"] -> w1040
                  frame False {
                  }
                  frame True {
                  }
                }
                n437 = Get Date/Time String() -> (date string=w1061:string, time string=w1062:string)  [unwired: 3 in]
                n438 = Concatenate Strings(w1061, w1062) -> (w1060:string)
                n439 = Number To Fractional String(number=w1048, precision (6)=i16 3) -> (F-format string=w1044:string)  [unwired: 2 in]
                n440 = Number To Fractional String(number=w1069, precision (6)=i16 3 ("width (-)")) -> (F-format string=w1059:string)  [unwired: 2 in]
                n441 = Number To Fractional String(number=w1067, precision (6)=i16 3 ("width (-)")) -> (F-format string=w1058:string)  [unwired: 2 in]
                n442 = Number To Fractional String(number=w1065, precision (6)=i16 3 ("width (-)")) -> (F-format string=w1057:string)  [unwired: 2 in]
                n443 = Number To Fractional String(number=w1046, precision (6)=i16 3) -> (F-format string=w1043:string)  [unwired: 2 in]
                n444 = Build Array(w1060, w1059, w1058, w1057, w1056, "1" ("element"), w1044, w1043, w1041, w1040) -> (w1054:string[])
                n445 = call-poly <vilib>:"Write Delimited Spreadsheet.vi"("file path (dialog if empty)"=w1050, "1D data"=w1054, "append to file? (new file:F)"=TRUE, "transpose? (no:F)"=FALSE, "delimiter (\\t)"="," ("delimiter (\\t)")) -> ()  [unwired: 9 in, 2 out]
              }
              frame 2 {
                n446 = case shown="True" w1076 {
                  tunnel: w1078 -> [_ w1083]
                  tunnel: w1077 -> [_ w1082]
                  tunnel: w1075 -> [_ w1081]
                  tunnel: w1074 -> [_ w1080]
                  frame False {
                  }
                  frame True {
                    n447 = Unbundle By Name(w1081) -> ("SET VALUE 1"=w1108:dbl, "TOL 1"=w1106:dbl, "RES VALUE 1"=w1104:dbl, "CH  PASS  1"=w1102:bool, "CH1 MAX TOL"=w1089:dbl, "CH1 MIN TOL"=w1087:dbl)
                    n448 = case shown="False" w1102 {
                      tunnel: ["FAIL" "PASS"] -> w1095
                      frame False {
                      }
                      frame True {
                      }
                    }
                    n449 = case shown="True" w1082 {
                      tunnel: ["NORMAL" "RETEST"] -> w1079
                      frame False {
                      }
                      frame True {
                      }
                    }
                    n450 = Get Date/Time String() -> (date string=w1100:string, time string=w1101:string)  [unwired: 3 in]
                    n451 = Concatenate Strings(w1100, w1101) -> (w1099:string)
                    n452 = Number To Fractional String(number=w1089, precision (6)=i16 3) -> (F-format string=w1085:string)  [unwired: 2 in]
                    n453 = Number To Fractional String(number=w1108, precision (6)=i16 3 ("width (-)")) -> (F-format string=w1098:string)  [unwired: 2 in]
                    n454 = Number To Fractional String(number=w1106, precision (6)=i16 3 ("width (-)")) -> (F-format string=w1097:string)  [unwired: 2 in]
                    n455 = Number To Fractional String(number=w1104, precision (6)=i16 3 ("width (-)")) -> (F-format string=w1096:string)  [unwired: 2 in]
                    n456 = Number To Fractional String(number=w1087, precision (6)=i16 3) -> (F-format string=w1084:string)  [unwired: 2 in]
                    n457 = Build Array(w1099, w1098, w1097, w1096, w1095, "1" ("element"), w1085, w1084, w1080, w1079) -> (w1093:string[])
                    n458 = call-poly <vilib>:"Write Delimited Spreadsheet.vi"("file path (dialog if empty)"=w1083, "1D data"=w1093, "append to file? (new file:F)"=TRUE, "transpose? (no:F)"=FALSE, "delimiter (\\t)"="," ("delimiter (\\t)")) -> ()  [unwired: 9 in, 2 out]
                  }
                }
              }
            }
          }
          frame #1 {
            # "CHANNEL 2 DATA LOG"
            n459 = Unbundle By Name(w1117) -> ("PP 2"=w1118:i32)
            n460 = case shown="1" w1118 {
              tunnel: w1117 -> [_ w1140 w1153]
              tunnel: w1113 -> [_ w1119 w1154]
              tunnel: w1116 -> [_ w1122 w1156]
              tunnel: w1115 -> [_ w1121 w1157]
              tunnel: w1114 -> [_ _ w1155]
              frame 0, Default {
              }
              frame 1 {
                n461 = Unbundle By Name(w1140) -> ("SET VALUE 2"=w1148:dbl, "TOL 2"=w1146:dbl, "RES VALUE 2"=w1144:dbl, "CH  PASS 2"=w1142:bool, "CH2 MAX TOL"=w1128:dbl, "CH2 MIN TOL"=w1127:dbl)
                n462 = case shown="False" w1142 {
                  tunnel: ["FAIL" "PASS"] -> w1134
                  frame False {
                  }
                  frame True {
                  }
                }
                n463 = case shown="True" w1122 {
                  tunnel: ["NORMAL" "RETEST"] -> w1120
                  frame False {
                  }
                  frame True {
                  }
                }
                n464 = Get Date/Time String() -> (date string=w1139:string, time string=w1141:string)  [unwired: 3 in]
                n465 = Concatenate Strings(w1139, w1141) -> (w1138:string)
                n466 = Number To Fractional String(number=w1128, precision (6)=i16 3) -> (F-format string=w1124:string)  [unwired: 2 in]
                n467 = Number To Fractional String(number=w1148, precision (6)=i16 3 ("width (-)")) -> (F-format string=w1137:string)  [unwired: 2 in]
                n468 = Number To Fractional String(number=w1146, precision (6)=i16 3 ("width (-)")) -> (F-format string=w1136:string)  [unwired: 2 in]
                n469 = Number To Fractional String(number=w1144, precision (6)=i16 3 ("width (-)")) -> (F-format string=w1135:string)  [unwired: 2 in]
                n470 = Number To Fractional String(number=w1127, precision (6)=i16 3) -> (F-format string=w1123:string)  [unwired: 2 in]
                n471 = Build Array(w1138, w1137, w1136, w1135, w1134, "2" ("element"), w1124, w1123, w1121, w1120) -> (w1132:string[])
                n472 = call-poly <vilib>:"Write Delimited Spreadsheet.vi"("file path (dialog if empty)"=w1119, "1D data"=w1132, "append to file? (new file:F)"=TRUE, "transpose? (no:F)"=FALSE, "delimiter (\\t)"="," ("delimiter (\\t)")) -> ()  [unwired: 9 in, 2 out]
              }
              frame 2 {
                n473 = case shown="False" w1155 {
                  tunnel: w1157 -> [_ w1161]
                  tunnel: w1156 -> [_ w1160]
                  tunnel: w1154 -> [_ w1159]
                  tunnel: w1153 -> [_ w1158]
                  frame False {
                  }
                  frame True {
                    n474 = Unbundle By Name(w1158) -> ("SET VALUE 2"=w1187:dbl, "TOL 2"=w1185:dbl, "RES VALUE 2"=w1183:dbl, "CH  PASS 2"=w1181:bool, "CH2 MAX TOL"=w1168:dbl, "CH2 MIN TOL"=w1167:dbl)
                    n475 = case shown="False" w1181 {
                      tunnel: ["FAIL" "PASS"] -> w1174
                      frame False {
                      }
                      frame True {
                      }
                    }
                    n476 = case shown="True" w1160 {
                      tunnel: ["NORMAL" "RETEST"] -> w1162
                      frame False {
                      }
                      frame True {
                      }
                    }
                    n477 = Get Date/Time String() -> (date string=w1179:string, time string=w1180:string)  [unwired: 3 in]
                    n478 = Concatenate Strings(w1179, w1180) -> (w1178:string)
                    n479 = Number To Fractional String(number=w1168, precision (6)=i16 3) -> (F-format string=w1164:string)  [unwired: 2 in]
                    n480 = Number To Fractional String(number=w1187, precision (6)=i16 3 ("width (-)")) -> (F-format string=w1177:string)  [unwired: 2 in]
                    n481 = Number To Fractional String(number=w1185, precision (6)=i16 3 ("width (-)")) -> (F-format string=w1176:string)  [unwired: 2 in]
                    n482 = Number To Fractional String(number=w1183, precision (6)=i16 3 ("width (-)")) -> (F-format string=w1175:string)  [unwired: 2 in]
                    n483 = Number To Fractional String(number=w1167, precision (6)=i16 3) -> (F-format string=w1163:string)  [unwired: 2 in]
                    n484 = Build Array(w1178, w1177, w1176, w1175, w1174, "2" ("element"), w1164, w1163, w1161, w1162) -> (w1172:string[])
                    n485 = call-poly <vilib>:"Write Delimited Spreadsheet.vi"("file path (dialog if empty)"=w1159, "1D data"=w1172, "append to file? (new file:F)"=TRUE, "transpose? (no:F)"=FALSE, "delimiter (\\t)"="," ("delimiter (\\t)")) -> ()  [unwired: 9 in, 2 out]
                  }
                }
              }
            }
          }
          frame #2 {
            # "Channel 3 data log"
            n486 = Unbundle By Name(w1196) -> ("PP 3"=w1197:i32)
            n487 = case shown="2" w1197 {
              tunnel: w1196 -> [_ w1207 w1232]
              tunnel: w1192 -> [_ w1208 w1236]
              tunnel: w1195 -> [_ w1200 w1234]
              tunnel: w1194 -> [_ w1199 w1235]
              tunnel: w1193 -> [_ _ w1233]
              frame 0, Default {
              }
              frame 1 {
                n488 = Unbundle By Name(w1207) -> ("SET VALUE 3"=w1227:dbl, "TOL 3"=w1225:dbl, "RES VALUE 3"=w1223:dbl, "CH  PASS 3"=w1221:bool, "CH3 MAX TOL"=w1206:dbl, "CH3 MIN TOL"=w1205:dbl)
                n489 = case shown="False" w1221 {
                  tunnel: ["FAIL" "PASS"] -> w1214
                  frame False {
                  }
                  frame True {
                  }
                }
                n490 = case shown="True" w1200 {
                  tunnel: ["NORMAL" "RETEST"] -> w1198
                  frame False {
                  }
                  frame True {
                  }
                }
                n491 = Get Date/Time String() -> (date string=w1219:string, time string=w1220:string)  [unwired: 3 in]
                n492 = Concatenate Strings(w1219, w1220) -> (w1218:string)
                n493 = Number To Fractional String(number=w1227, precision (6)=i16 3 ("width (-)")) -> (F-format string=w1217:string)  [unwired: 2 in]
                n494 = Number To Fractional String(number=w1225, precision (6)=i16 3 ("width (-)")) -> (F-format string=w1216:string)  [unwired: 2 in]
                n495 = Number To Fractional String(number=w1223, precision (6)=i16 3 ("width (-)")) -> (F-format string=w1215:string)  [unwired: 2 in]
                n496 = Number To Fractional String(number=w1206, precision (6)=i16 3) -> (F-format string=w1202:string)  [unwired: 2 in]
                n497 = Number To Fractional String(number=w1205, precision (6)=i16 3) -> (F-format string=w1201:string)  [unwired: 2 in]
                n498 = Build Array(w1218, w1217, w1216, w1215, w1214, "3" ("element"), w1202, w1201, w1199, w1198) -> (w1212:string[])
                n499 = call-poly <vilib>:"Write Delimited Spreadsheet.vi"("file path (dialog if empty)"=w1208, "1D data"=w1212, "append to file? (new file:F)"=TRUE, "transpose? (no:F)"=FALSE, "delimiter (\\t)"="," ("delimiter (\\t)")) -> ()  [unwired: 9 in, 2 out]
              }
              frame 2 {
                n500 = case shown="True" w1233 {
                  tunnel: w1236 -> [_ w1240]
                  tunnel: w1235 -> [_ w1239]
                  tunnel: w1234 -> [_ w1238]
                  tunnel: w1232 -> [_ w1237]
                  frame False {
                  }
                  frame True {
                    n501 = Unbundle By Name(w1237) -> ("SET VALUE 3"=w1266:dbl, "TOL 3"=w1264:dbl, "RES VALUE 3"=w1262:dbl, "CH  PASS 3"=w1260:bool, "CH3 MAX TOL"=w1247:dbl, "CH3 MIN TOL"=w1246:dbl)
                    n502 = case shown="False" w1260 {
                      tunnel: ["FAIL" "PASS"] -> w1253
                      frame False {
                      }
                      frame True {
                      }
                    }
                    n503 = case shown="True" w1238 {
                      tunnel: ["NORMAL" "RETEST"] -> w1241
                      frame False {
                      }
                      frame True {
                      }
                    }
                    n504 = Get Date/Time String() -> (date string=w1258:string, time string=w1259:string)  [unwired: 3 in]
                    n505 = Concatenate Strings(w1258, w1259) -> (w1257:string)
                    n506 = Number To Fractional String(number=w1266, precision (6)=i16 3 ("width (-)")) -> (F-format string=w1256:string)  [unwired: 2 in]
                    n507 = Number To Fractional String(number=w1264, precision (6)=i16 3 ("width (-)")) -> (F-format string=w1255:string)  [unwired: 2 in]
                    n508 = Number To Fractional String(number=w1262, precision (6)=i16 3 ("width (-)")) -> (F-format string=w1254:string)  [unwired: 2 in]
                    n509 = Number To Fractional String(number=w1247, precision (6)=i16 3) -> (F-format string=w1243:string)  [unwired: 2 in]
                    n510 = Number To Fractional String(number=w1246, precision (6)=i16 3) -> (F-format string=w1242:string)  [unwired: 2 in]
                    n511 = Build Array(w1257, w1256, w1255, w1254, w1253, "3" ("element"), w1243, w1242, w1239, w1241) -> (w1251:string[])
                    n512 = call-poly <vilib>:"Write Delimited Spreadsheet.vi"("file path (dialog if empty)"=w1240, "1D data"=w1251, "append to file? (new file:F)"=TRUE, "transpose? (no:F)"=FALSE, "delimiter (\\t)"="," ("delimiter (\\t)")) -> ()  [unwired: 9 in, 2 out]
                  }
                }
              }
            }
          }
          frame #3 {
            # "Channel 4 data log"
            n513 = Unbundle By Name(w1275) -> ("PP 4"=w1276:i32)
            n514 = case shown="2" w1276 {
              tunnel: w1275 -> [_ w1286 w1312]
              tunnel: w1271 -> [_ w1287 w1313]
              tunnel: w1274 -> [_ w1279 w1314]
              tunnel: w1273 -> [_ w1278 w1315]
              tunnel: w1272 -> [_ _ w1311]
              frame 0, Default {
              }
              frame 1 {
                n515 = Unbundle By Name(w1286) -> ("SET VALUE 4"=w1306:dbl, "TOL 4"=w1304:dbl, "RES VALUE 4"=w1302:dbl, "CH  PASS 4"=w1300:bool, "CH4 MAX TOL"=w1285:dbl, "CH4 MIN TOL"=w1282:dbl)
                n516 = case shown="False" w1300 {
                  tunnel: ["FAIL" "PASS"] -> w1293
                  frame False {
                  }
                  frame True {
                  }
                }
                n517 = case shown="True" w1279 {
                  tunnel: ["NORMAL" "RETEST"] -> w1277
                  frame False {
                  }
                  frame True {
                  }
                }
                n518 = Get Date/Time String() -> (date string=w1298:string, time string=w1299:string)  [unwired: 3 in]
                n519 = Concatenate Strings(w1298, w1299) -> (w1297:string)
                n520 = Number To Fractional String(number=w1282, precision (6)=i16 3) -> (F-format string=w1280:string)  [unwired: 2 in]
                n521 = Number To Fractional String(number=w1306, precision (6)=i16 3 ("width (-)")) -> (F-format string=w1296:string)  [unwired: 2 in]
                n522 = Number To Fractional String(number=w1304, precision (6)=i16 3 ("width (-)")) -> (F-format string=w1295:string)  [unwired: 2 in]
                n523 = Number To Fractional String(number=w1302, precision (6)=i16 3 ("width (-)")) -> (F-format string=w1294:string)  [unwired: 2 in]
                n524 = Number To Fractional String(number=w1285, precision (6)=i16 3) -> (F-format string=w1283:string)  [unwired: 2 in]
                n525 = Build Array(w1297, w1296, w1295, w1294, w1293, "4" ("element"), w1283, w1280, w1278, w1277) -> (w1291:string[])
                n526 = call-poly <vilib>:"Write Delimited Spreadsheet.vi"("file path (dialog if empty)"=w1287, "1D data"=w1291, "append to file? (new file:F)"=TRUE, "transpose? (no:F)"=FALSE, "delimiter (\\t)"="," ("delimiter (\\t)")) -> ()  [unwired: 9 in, 2 out]
              }
              frame 2 {
                n527 = case shown="True" w1311 {
                  tunnel: w1315 -> [_ w1319]
                  tunnel: w1314 -> [_ w1318]
                  tunnel: w1313 -> [_ w1317]
                  tunnel: w1312 -> [_ w1316]
                  frame False {
                  }
                  frame True {
                    n528 = Unbundle By Name(w1316) -> ("SET VALUE 4"=w1345:dbl, "TOL 4"=w1343:dbl, "RES VALUE 4"=w1341:dbl, "CH  PASS 4"=w1339:bool, "CH4 MAX TOL"=w1326:dbl, "CH4 MIN TOL"=w1323:dbl)
                    n529 = case shown="False" w1339 {
                      tunnel: ["FAIL" "PASS"] -> w1332
                      frame False {
                      }
                      frame True {
                      }
                    }
                    n530 = case shown="True" w1318 {
                      tunnel: ["NORMAL" "RETEST"] -> w1320
                      frame False {
                      }
                      frame True {
                      }
                    }
                    n531 = Get Date/Time String() -> (date string=w1337:string, time string=w1338:string)  [unwired: 3 in]
                    n532 = Concatenate Strings(w1337, w1338) -> (w1336:string)
                    n533 = Number To Fractional String(number=w1323, precision (6)=i16 3) -> (F-format string=w1321:string)  [unwired: 2 in]
                    n534 = Number To Fractional String(number=w1345, precision (6)=i16 3 ("width (-)")) -> (F-format string=w1335:string)  [unwired: 2 in]
                    n535 = Number To Fractional String(number=w1343, precision (6)=i16 3 ("width (-)")) -> (F-format string=w1334:string)  [unwired: 2 in]
                    n536 = Number To Fractional String(number=w1341, precision (6)=i16 3 ("width (-)")) -> (F-format string=w1333:string)  [unwired: 2 in]
                    n537 = Number To Fractional String(number=w1326, precision (6)=i16 3) -> (F-format string=w1324:string)  [unwired: 2 in]
                    n538 = Build Array(w1336, w1335, w1334, w1333, w1332, "4" ("element"), w1324, w1321, w1319, w1320) -> (w1330:string[])
                    n539 = call-poly <vilib>:"Write Delimited Spreadsheet.vi"("file path (dialog if empty)"=w1317, "1D data"=w1330, "append to file? (new file:F)"=TRUE, "transpose? (no:F)"=FALSE, "delimiter (\\t)"="," ("delimiter (\\t)")) -> ()  [unwired: 9 in, 2 out]
                  }
                }
              }
            }
          }
          frame #4 {
            # "Channel 5 data log"
            n540 = Unbundle By Name(w1354) -> ("PP 5"=w1355:i32)
            n541 = case shown="1" w1355 {
              tunnel: w1354 -> [_ w1365 w1391]
              tunnel: w1350 -> [_ w1366 w1392]
              tunnel: w1353 -> [_ w1360 w1393]
              tunnel: w1352 -> [_ w1357 w1394]
              tunnel: w1351 -> [_ _ w1390]
              frame 0, Default {
              }
              frame 1 {
                n542 = Unbundle By Name(w1365) -> ("SET VALUE 5"=w1385:dbl, "TOL 5"=w1383:dbl, "RES VALUE 5"=w1381:dbl, "CH  PASS 5"=w1379:bool, "CH5 MAX TOL"=w1364:dbl, "CH5 MIN TOL"=w1362:dbl)
                n543 = case shown="False" w1379 {
                  tunnel: ["FAIL" "PASS"] -> w1372
                  frame False {
                  }
                  frame True {
                  }
                }
                n544 = case shown="True" w1360 {
                  tunnel: ["NORMAL" "RETEST"] -> w1356
                  frame False {
                  }
                  frame True {
                  }
                }
                n545 = Get Date/Time String() -> (date string=w1377:string, time string=w1378:string)  [unwired: 3 in]
                n546 = Concatenate Strings(w1377, w1378) -> (w1376:string)
                n547 = Number To Fractional String(number=w1385, precision (6)=i16 3 ("width (-)")) -> (F-format string=w1375:string)  [unwired: 2 in]
                n548 = Number To Fractional String(number=w1383, precision (6)=i16 3 ("width (-)")) -> (F-format string=w1374:string)  [unwired: 2 in]
                n549 = Number To Fractional String(number=w1381, precision (6)=i16 3 ("width (-)")) -> (F-format string=w1373:string)  [unwired: 2 in]
                n550 = Number To Fractional String(number=w1364, precision (6)=i16 3) -> (F-format string=w1359:string)  [unwired: 2 in]
                n551 = Number To Fractional String(number=w1362, precision (6)=i16 3) -> (F-format string=w1358:string)  [unwired: 2 in]
                n552 = Build Array(w1376, w1375, w1374, w1373, w1372, "5" ("element"), w1359, w1358, w1357, w1356) -> (w1370:string[])
                n553 = call-poly <vilib>:"Write Delimited Spreadsheet.vi"("file path (dialog if empty)"=w1366, "1D data"=w1370, "append to file? (new file:F)"=TRUE, "transpose? (no:F)"=FALSE, "delimiter (\\t)"="," ("delimiter (\\t)")) -> ()  [unwired: 9 in, 2 out]
              }
              frame 2 {
                n554 = case shown="True" w1390 {
                  tunnel: w1394 -> [_ w1398]
                  tunnel: w1393 -> [_ w1397]
                  tunnel: w1392 -> [_ w1396]
                  tunnel: w1391 -> [_ w1395]
                  frame False {
                  }
                  frame True {
                    n555 = Unbundle By Name(w1395) -> ("SET VALUE 5"=w1424:dbl, "TOL 5"=w1422:dbl, "RES VALUE 5"=w1420:dbl, "CH  PASS 5"=w1418:bool, "CH5 MAX TOL"=w1405:dbl, "CH5 MIN TOL"=w1403:dbl)
                    n556 = case shown="False" w1418 {
                      tunnel: ["FAIL" "PASS"] -> w1411
                      frame False {
                      }
                      frame True {
                      }
                    }
                    n557 = case shown="True" w1397 {
                      tunnel: ["NORMAL" "RETEST"] -> w1399
                      frame False {
                      }
                      frame True {
                      }
                    }
                    n558 = Get Date/Time String() -> (date string=w1416:string, time string=w1417:string)  [unwired: 3 in]
                    n559 = Concatenate Strings(w1416, w1417) -> (w1415:string)
                    n560 = Number To Fractional String(number=w1424, precision (6)=i16 3 ("width (-)")) -> (F-format string=w1414:string)  [unwired: 2 in]
                    n561 = Number To Fractional String(number=w1422, precision (6)=i16 3 ("width (-)")) -> (F-format string=w1413:string)  [unwired: 2 in]
                    n562 = Number To Fractional String(number=w1420, precision (6)=i16 3 ("width (-)")) -> (F-format string=w1412:string)  [unwired: 2 in]
                    n563 = Number To Fractional String(number=w1405, precision (6)=i16 3) -> (F-format string=w1401:string)  [unwired: 2 in]
                    n564 = Number To Fractional String(number=w1403, precision (6)=i16 3) -> (F-format string=w1400:string)  [unwired: 2 in]
                    n565 = Build Array(w1415, w1414, w1413, w1412, w1411, "5" ("element"), w1401, w1400, w1398, w1399) -> (w1409:string[])
                    n566 = call-poly <vilib>:"Write Delimited Spreadsheet.vi"("file path (dialog if empty)"=w1396, "1D data"=w1409, "append to file? (new file:F)"=TRUE, "transpose? (no:F)"=FALSE, "delimiter (\\t)"="," ("delimiter (\\t)")) -> ()  [unwired: 9 in, 2 out]
                  }
                }
              }
            }
          }
          frame #5 {
            # "Channel 6 data log"
            n567 = Unbundle By Name(w1433) -> ("PP 6"=w1434:i32)
            n568 = case shown="1" w1434 {
              tunnel: w1433 -> [_ w1444 w1470]
              tunnel: w1429 -> [_ w1445 w1471]
              tunnel: w1432 -> [_ w1437 w1473]
              tunnel: w1431 -> [_ w1436 w1472]
              tunnel: w1430 -> [_ _ w1469]
              frame 0, Default {
              }
              frame 1 {
                n569 = Unbundle By Name(w1444) -> ("SET VALUE 6"=w1464:dbl, "TOL 6"=w1462:dbl, "RES VALUE 6"=w1460:dbl, "CH  PASS 6"=w1458:bool, "CH6 MAX TOL"=w1441:dbl, "CH6 MIN TOL"=w1440:dbl)
                n570 = case shown="False" w1458 {
                  tunnel: ["FAIL" "PASS"] -> w1451
                  frame False {
                  }
                  frame True {
                  }
                }
                n571 = case shown="True" w1437 {
                  tunnel: ["NORMAL" "RETEST"] -> w1435
                  frame False {
                  }
                  frame True {
                  }
                }
                n572 = Get Date/Time String() -> (date string=w1456:string, time string=w1457:string)  [unwired: 3 in]
                n573 = Concatenate Strings(w1456, w1457) -> (w1455:string)
                n574 = Number To Fractional String(number=w1464, precision (6)=i16 3 ("width (-)")) -> (F-format string=w1454:string)  [unwired: 2 in]
                n575 = Number To Fractional String(number=w1462, precision (6)=i16 3 ("width (-)")) -> (F-format string=w1453:string)  [unwired: 2 in]
                n576 = Number To Fractional String(number=w1460, precision (6)=i16 3 ("width (-)")) -> (F-format string=w1452:string)  [unwired: 2 in]
                n577 = Number To Fractional String(number=w1441, precision (6)=i16 3) -> (F-format string=w1439:string)  [unwired: 2 in]
                n578 = Number To Fractional String(number=w1440, precision (6)=i16 3) -> (F-format string=w1438:string)  [unwired: 2 in]
                n579 = Build Array(w1455, w1454, w1453, w1452, w1451, "6" ("element"), w1439, w1438, w1436, w1435) -> (w1449:string[])
                n580 = call-poly <vilib>:"Write Delimited Spreadsheet.vi"("file path (dialog if empty)"=w1445, "1D data"=w1449, "append to file? (new file:F)"=TRUE, "transpose? (no:F)"=FALSE, "delimiter (\\t)"="," ("delimiter (\\t)")) -> ()  [unwired: 9 in, 2 out]
              }
              frame 2 {
                n581 = case shown="True" w1469 {
                  tunnel: w1473 -> [_ w1477]
                  tunnel: w1472 -> [_ w1476]
                  tunnel: w1471 -> [_ w1475]
                  tunnel: w1470 -> [_ w1474]
                  frame False {
                  }
                  frame True {
                    n582 = Unbundle By Name(w1474) -> ("SET VALUE 6"=w1503:dbl, "TOL 6"=w1501:dbl, "RES VALUE 6"=w1499:dbl, "CH  PASS 6"=w1497:bool, "CH6 MAX TOL"=w1482:dbl, "CH6 MIN TOL"=w1481:dbl)
                    n583 = case shown="False" w1497 {
                      tunnel: ["FAIL" "PASS"] -> w1490
                      frame False {
                      }
                      frame True {
                      }
                    }
                    n584 = case shown="True" w1477 {
                      tunnel: ["NORMAL" "RETEST"] -> w1478
                      frame False {
                      }
                      frame True {
                      }
                    }
                    n585 = Get Date/Time String() -> (date string=w1495:string, time string=w1496:string)  [unwired: 3 in]
                    n586 = Concatenate Strings(w1495, w1496) -> (w1494:string)
                    n587 = Number To Fractional String(number=w1503, precision (6)=i16 3 ("width (-)")) -> (F-format string=w1493:string)  [unwired: 2 in]
                    n588 = Number To Fractional String(number=w1501, precision (6)=i16 3 ("width (-)")) -> (F-format string=w1492:string)  [unwired: 2 in]
                    n589 = Number To Fractional String(number=w1499, precision (6)=i16 3 ("width (-)")) -> (F-format string=w1491:string)  [unwired: 2 in]
                    n590 = Number To Fractional String(number=w1482, precision (6)=i16 3) -> (F-format string=w1480:string)  [unwired: 2 in]
                    n591 = Number To Fractional String(number=w1481, precision (6)=i16 3) -> (F-format string=w1479:string)  [unwired: 2 in]
                    n592 = Build Array(w1494, w1493, w1492, w1491, w1490, "6" ("element"), w1480, w1479, w1476, w1478) -> (w1488:string[])
                    n593 = call-poly <vilib>:"Write Delimited Spreadsheet.vi"("file path (dialog if empty)"=w1475, "1D data"=w1488, "append to file? (new file:F)"=TRUE, "transpose? (no:F)"=FALSE, "delimiter (\\t)"="," ("delimiter (\\t)")) -> ()  [unwired: 9 in, 2 out]
                  }
                }
              }
            }
          }
          frame #6 {
            # "Channel 7 data log"
            n594 = Unbundle By Name(w1512) -> ("PP 7"=w1513:i32)
            n595 = case shown="1" w1513 {
              tunnel: w1512 -> [_ w1523 w1548]
              tunnel: w1508 -> [_ w1524 w1551]
              tunnel: w1511 -> [_ w1516 w1549]
              tunnel: w1510 -> [_ w1515 w1550]
              tunnel: w1509 -> [_ _ w1552]
              frame 0, Default {
              }
              frame 1 {
                n596 = Unbundle By Name(w1523) -> ("SET VALUE 7"=w1543:dbl, "TOL 7"=w1541:dbl, "RES VALUE 7"=w1539:dbl, "CH  PASS 7"=w1537:bool, "CH7 MAX TOL"=w1522:dbl, "CH7 MIN TOL"=w1520:dbl)
                n597 = case shown="False" w1537 {
                  tunnel: ["FAIL" "PASS"] -> w1530
                  frame False {
                  }
                  frame True {
                  }
                }
                n598 = case shown="False" w1516 {
                  tunnel: ["NORMAL" "RETEST"] -> w1514
                  frame False {
                  }
                  frame True {
                  }
                }
                n599 = Get Date/Time String() -> (date string=w1535:string, time string=w1536:string)  [unwired: 3 in]
                n600 = Concatenate Strings(w1535, w1536) -> (w1534:string)
                n601 = Number To Fractional String(number=w1543, precision (6)=i16 3 ("width (-)")) -> (F-format string=w1533:string)  [unwired: 2 in]
                n602 = Number To Fractional String(number=w1541, precision (6)=i16 3 ("width (-)")) -> (F-format string=w1532:string)  [unwired: 2 in]
                n603 = Number To Fractional String(number=w1539, precision (6)=i16 3 ("width (-)")) -> (F-format string=w1531:string)  [unwired: 2 in]
                n604 = Number To Fractional String(number=w1522, precision (6)=i16 3) -> (F-format string=w1518:string)  [unwired: 2 in]
                n605 = Number To Fractional String(number=w1520, precision (6)=i16 3) -> (F-format string=w1517:string)  [unwired: 2 in]
                n606 = Build Array(w1534, w1533, w1532, w1531, w1530, "7" ("element"), w1518, w1517, w1515, w1514) -> (w1528:string[])
                n607 = call-poly <vilib>:"Write Delimited Spreadsheet.vi"("file path (dialog if empty)"=w1524, "1D data"=w1528, "append to file? (new file:F)"=TRUE, "transpose? (no:F)"=FALSE, "delimiter (\\t)"="," ("delimiter (\\t)")) -> ()  [unwired: 9 in, 2 out]
              }
              frame 2 {
                n608 = case shown="True" w1552 {
                  tunnel: w1551 -> [_ w1556]
                  tunnel: w1550 -> [_ w1555]
                  tunnel: w1549 -> [_ w1554]
                  tunnel: w1548 -> [_ w1553]
                  frame False {
                  }
                  frame True {
                    n609 = Unbundle By Name(w1553) -> ("SET VALUE 7"=w1582:dbl, "TOL 7"=w1580:dbl, "RES VALUE 7"=w1578:dbl, "CH  PASS 7"=w1576:bool, "CH7 MAX TOL"=w1563:dbl, "CH7 MIN TOL"=w1561:dbl)
                    n610 = case shown="False" w1576 {
                      tunnel: ["FAIL" "PASS"] -> w1569
                      frame False {
                      }
                      frame True {
                      }
                    }
                    n611 = case shown="False" w1554 {
                      tunnel: ["NORMAL" "RETEST"] -> w1557
                      frame False {
                      }
                      frame True {
                      }
                    }
                    n612 = Get Date/Time String() -> (date string=w1574:string, time string=w1575:string)  [unwired: 3 in]
                    n613 = Concatenate Strings(w1574, w1575) -> (w1573:string)
                    n614 = Number To Fractional String(number=w1582, precision (6)=i16 3 ("width (-)")) -> (F-format string=w1572:string)  [unwired: 2 in]
                    n615 = Number To Fractional String(number=w1580, precision (6)=i16 3 ("width (-)")) -> (F-format string=w1571:string)  [unwired: 2 in]
                    n616 = Number To Fractional String(number=w1578, precision (6)=i16 3 ("width (-)")) -> (F-format string=w1570:string)  [unwired: 2 in]
                    n617 = Number To Fractional String(number=w1563, precision (6)=i16 3) -> (F-format string=w1559:string)  [unwired: 2 in]
                    n618 = Number To Fractional String(number=w1561, precision (6)=i16 3) -> (F-format string=w1558:string)  [unwired: 2 in]
                    n619 = Build Array(w1573, w1572, w1571, w1570, w1569, "7" ("element"), w1559, w1558, w1555, w1557) -> (w1567:string[])
                    n620 = call-poly <vilib>:"Write Delimited Spreadsheet.vi"("file path (dialog if empty)"=w1556, "1D data"=w1567, "append to file? (new file:F)"=TRUE, "transpose? (no:F)"=FALSE, "delimiter (\\t)"="," ("delimiter (\\t)")) -> ()  [unwired: 9 in, 2 out]
                  }
                }
              }
            }
          }
          frame #7 {
            # "Channel 8 data log"
            n621 = Unbundle By Name(w1591) -> ("PP 8"=w1592:i32)
            n622 = case shown="2" w1592 {
              tunnel: w1591 -> [_ w1602 w1630]
              tunnel: w1587 -> [_ w1603 w1631]
              tunnel: w1590 -> [_ w1597 w1628]
              tunnel: w1589 -> [_ w1594 w1629]
              tunnel: w1588 -> [_ _ w1627]
              frame 0, Default {
              }
              frame 1 {
                n623 = Unbundle By Name(w1602) -> ("SET VALUE 8"=w1622:dbl, "TOL 8"=w1620:dbl, "RES VALUE 8"=w1618:dbl, "CH  PASS 8"=w1616:bool, "CH8 MAX TOL"=w1601:dbl, "CH8 MIN TOL"=w1599:dbl)
                n624 = case shown="False" w1616 {
                  tunnel: ["FAIL" "PASS"] -> w1609
                  frame False {
                  }
                  frame True {
                  }
                }
                n625 = case shown="True" w1597 {
                  tunnel: ["NORMAL" "RETEST"] -> w1593
                  frame False {
                  }
                  frame True {
                  }
                }
                n626 = Get Date/Time String() -> (date string=w1614:string, time string=w1615:string)  [unwired: 3 in]
                n627 = Concatenate Strings(w1614, w1615) -> (w1613:string)
                n628 = Number To Fractional String(number=w1601, precision (6)=i16 3) -> (F-format string=w1596:string)  [unwired: 2 in]
                n629 = Number To Fractional String(number=w1622, precision (6)=i16 3 ("width (-)")) -> (F-format string=w1612:string)  [unwired: 2 in]
                n630 = Number To Fractional String(number=w1620, precision (6)=i16 3 ("width (-)")) -> (F-format string=w1611:string)  [unwired: 2 in]
                n631 = Number To Fractional String(number=w1618, precision (6)=i16 3 ("width (-)")) -> (F-format string=w1610:string)  [unwired: 2 in]
                n632 = Number To Fractional String(number=w1599, precision (6)=i16 3) -> (F-format string=w1595:string)  [unwired: 2 in]
                n633 = Build Array(w1613, w1612, w1611, w1610, w1609, "8" ("element"), w1596, w1595, w1594, w1593) -> (w1607:string[])
                n634 = call-poly <vilib>:"Write Delimited Spreadsheet.vi"("file path (dialog if empty)"=w1603, "1D data"=w1607, "append to file? (new file:F)"=TRUE, "transpose? (no:F)"=FALSE, "delimiter (\\t)"="," ("delimiter (\\t)")) -> ()  [unwired: 9 in, 2 out]
              }
              frame 2 {
                n635 = case shown="True" w1627 {
                  tunnel: w1631 -> [_ w1635]
                  tunnel: w1630 -> [_ w1634]
                  tunnel: w1629 -> [_ w1633]
                  tunnel: w1628 -> [_ w1632]
                  frame False {
                  }
                  frame True {
                    n636 = Unbundle By Name(w1634) -> ("SET VALUE 8"=w1661:dbl, "TOL 8"=w1659:dbl, "RES VALUE 8"=w1657:dbl, "CH  PASS 8"=w1655:bool, "CH8 MAX TOL"=w1642:dbl, "CH8 MIN TOL"=w1640:dbl)
                    n637 = case shown="False" w1655 {
                      tunnel: ["FAIL" "PASS"] -> w1648
                      frame False {
                      }
                      frame True {
                      }
                    }
                    n638 = case shown="True" w1632 {
                      tunnel: ["NORMAL" "RETEST"] -> w1636
                      frame False {
                      }
                      frame True {
                      }
                    }
                    n639 = Get Date/Time String() -> (date string=w1653:string, time string=w1654:string)  [unwired: 3 in]
                    n640 = Concatenate Strings(w1653, w1654) -> (w1652:string)
                    n641 = Number To Fractional String(number=w1642, precision (6)=i16 3) -> (F-format string=w1638:string)  [unwired: 2 in]
                    n642 = Number To Fractional String(number=w1661, precision (6)=i16 3 ("width (-)")) -> (F-format string=w1651:string)  [unwired: 2 in]
                    n643 = Number To Fractional String(number=w1659, precision (6)=i16 3 ("width (-)")) -> (F-format string=w1650:string)  [unwired: 2 in]
                    n644 = Number To Fractional String(number=w1657, precision (6)=i16 3 ("width (-)")) -> (F-format string=w1649:string)  [unwired: 2 in]
                    n645 = Number To Fractional String(number=w1640, precision (6)=i16 3) -> (F-format string=w1637:string)  [unwired: 2 in]
                    n646 = Build Array(w1652, w1651, w1650, w1649, w1648, "8" ("element"), w1638, w1637, w1633, w1636) -> (w1646:string[])
                    n647 = call-poly <vilib>:"Write Delimited Spreadsheet.vi"("file path (dialog if empty)"=w1635, "1D data"=w1646, "append to file? (new file:F)"=TRUE, "transpose? (no:F)"=FALSE, "delimiter (\\t)"="," ("delimiter (\\t)")) -> ()  [unwired: 9 in, 2 out]
                  }
                }
              }
            }
          }
          frame #8 {
            # "Channel 9 data log"
            n648 = Unbundle By Name(w1670) -> ("PP 9"=w1671:i32)
            n649 = case shown="1" w1671 {
              tunnel: w1670 -> [_ w1682 w1707]
              tunnel: w1669 -> [_ w1675 w1708]
              tunnel: w1668 -> [_ w1673 w1709]
              tunnel: w1667 -> [_ _ w1710]
              tunnel: w1666 -> [_ w1672 w1706]
              frame 0, Default {
              }
              frame 1 {
                n650 = Unbundle By Name(w1682) -> ("SET VALUE 9"=w1701:dbl, "TOL 9"=w1699:dbl, "RES VALUE 9"=w1697:dbl, "CH  PASS 9"=w1695:bool, "CH9 MAX TOL"=w1681:dbl, "CH9 MIN TOL"=w1680:dbl)
                n651 = case shown="False" w1695 {
                  tunnel: ["FAIL" "PASS"] -> w1688
                  frame False {
                  }
                  frame True {
                  }
                }
                n652 = case shown="False" w1675 {
                  tunnel: ["NORMAL" "RETEST"] -> w1674
                  frame False {
                  }
                  frame True {
                  }
                }
                n653 = Get Date/Time String() -> (date string=w1693:string, time string=w1694:string)  [unwired: 3 in]
                n654 = Concatenate Strings(w1693, w1694) -> (w1692:string)
                n655 = Number To Fractional String(number=w1681, precision (6)=i16 3) -> (F-format string=w1677:string)  [unwired: 2 in]
                n656 = Number To Fractional String(number=w1701, precision (6)=i16 3 ("width (-)")) -> (F-format string=w1691:string)  [unwired: 2 in]
                n657 = Number To Fractional String(number=w1699, precision (6)=i16 3 ("width (-)")) -> (F-format string=w1690:string)  [unwired: 2 in]
                n658 = Number To Fractional String(number=w1697, precision (6)=i16 3 ("width (-)")) -> (F-format string=w1689:string)  [unwired: 2 in]
                n659 = Number To Fractional String(number=w1680, precision (6)=i16 3) -> (F-format string=w1676:string)  [unwired: 2 in]
                n660 = Build Array(w1692, w1691, w1690, w1689, w1688, "9" ("element"), w1677, w1676, w1673, w1674) -> (w1686:string[])
                n661 = call-poly <vilib>:"Write Delimited Spreadsheet.vi"("file path (dialog if empty)"=w1672, "1D data"=w1686, "append to file? (new file:F)"=TRUE, "transpose? (no:F)"=FALSE, "delimiter (\\t)"="," ("delimiter (\\t)")) -> ()  [unwired: 9 in, 2 out]
              }
              frame 2 {
                n662 = case shown="True" w1710 {
                  tunnel: w1706 -> [_ w1714]
                  tunnel: w1709 -> [_ w1713]
                  tunnel: w1708 -> [_ w1712]
                  tunnel: w1707 -> [_ w1711]
                  frame False {
                  }
                  frame True {
                    n663 = Unbundle By Name(w1711) -> ("SET VALUE 9"=w1740:dbl, "TOL 9"=w1738:dbl, "RES VALUE 9"=w1736:dbl, "CH  PASS 9"=w1734:bool, "CH9 MAX TOL"=w1721:dbl, "CH9 MIN TOL"=w1720:dbl)
                    n664 = case shown="False" w1734 {
                      tunnel: ["FAIL" "PASS"] -> w1727
                      frame False {
                      }
                      frame True {
                      }
                    }
                    n665 = case shown="False" w1712 {
                      tunnel: ["NORMAL" "RETEST"] -> w1715
                      frame False {
                      }
                      frame True {
                      }
                    }
                    n666 = Get Date/Time String() -> (date string=w1732:string, time string=w1733:string)  [unwired: 3 in]
                    n667 = Concatenate Strings(w1732, w1733) -> (w1731:string)
                    n668 = Number To Fractional String(number=w1721, precision (6)=i16 3) -> (F-format string=w1717:string)  [unwired: 2 in]
                    n669 = Number To Fractional String(number=w1740, precision (6)=i16 3 ("width (-)")) -> (F-format string=w1730:string)  [unwired: 2 in]
                    n670 = Number To Fractional String(number=w1738, precision (6)=i16 3 ("width (-)")) -> (F-format string=w1729:string)  [unwired: 2 in]
                    n671 = Number To Fractional String(number=w1736, precision (6)=i16 3 ("width (-)")) -> (F-format string=w1728:string)  [unwired: 2 in]
                    n672 = Number To Fractional String(number=w1720, precision (6)=i16 3) -> (F-format string=w1716:string)  [unwired: 2 in]
                    n673 = Build Array(w1731, w1730, w1729, w1728, w1727, "9" ("element"), w1717, w1716, w1713, w1715) -> (w1725:string[])
                    n674 = call-poly <vilib>:"Write Delimited Spreadsheet.vi"("file path (dialog if empty)"=w1714, "1D data"=w1725, "append to file? (new file:F)"=TRUE, "transpose? (no:F)"=FALSE, "delimiter (\\t)"="," ("delimiter (\\t)")) -> ()  [unwired: 9 in, 2 out]
                  }
                }
              }
            }
          }
          frame #9 {
            # "Channel 10 data log"
            n675 = Unbundle By Name(w1749) -> ("PP 10"=w1750:i32)
            n676 = case shown="2" w1750 {
              tunnel: w1749 -> [_ w1760 w1788]
              tunnel: w1745 -> [_ w1761 w1789]
              tunnel: w1748 -> [_ w1755 w1786]
              tunnel: w1747 -> [_ w1752 w1787]
              tunnel: w1746 -> [_ _ w1785]
              frame 0, Default {
              }
              frame 1 {
                n677 = Unbundle By Name(w1760) -> ("SET VALUE 10"=w1780:dbl, "TOL 10"=w1778:dbl, "RES VALUE 10"=w1776:dbl, "CH  PASS 10"=w1774:bool, "CH10 MAX TOL"=w1759:dbl, "CH10 MIN TOL"=w1758:dbl)
                n678 = case shown="False" w1774 {
                  tunnel: ["FAIL" "PASS"] -> w1767
                  frame False {
                  }
                  frame True {
                  }
                }
                n679 = case shown="True" w1755 {
                  tunnel: ["NORMAL" "RETEST"] -> w1751
                  frame False {
                  }
                  frame True {
                  }
                }
                n680 = Get Date/Time String() -> (date string=w1772:string, time string=w1773:string)  [unwired: 3 in]
                n681 = Concatenate Strings(w1772, w1773) -> (w1771:string)
                n682 = Number To Fractional String(number=w1759, precision (6)=i16 3) -> (F-format string=w1757:string)  [unwired: 2 in]
                n683 = Number To Fractional String(number=w1780, precision (6)=i16 3 ("width (-)")) -> (F-format string=w1770:string)  [unwired: 2 in]
                n684 = Number To Fractional String(number=w1778, precision (6)=i16 3 ("width (-)")) -> (F-format string=w1769:string)  [unwired: 2 in]
                n685 = Number To Fractional String(number=w1776, precision (6)=i16 3 ("width (-)")) -> (F-format string=w1768:string)  [unwired: 2 in]
                n686 = Number To Fractional String(number=w1758, precision (6)=i16 3) -> (F-format string=w1756:string)  [unwired: 2 in]
                n687 = Build Array(w1771, w1770, w1769, w1768, w1767, "10" ("element"), w1757, w1756, w1752, w1751) -> (w1765:string[])
                n688 = call-poly <vilib>:"Write Delimited Spreadsheet.vi"("file path (dialog if empty)"=w1761, "1D data"=w1765, "append to file? (new file:F)"=TRUE, "transpose? (no:F)"=FALSE, "delimiter (\\t)"="," ("delimiter (\\t)")) -> ()  [unwired: 9 in, 2 out]
              }
              frame 2 {
                n689 = case shown="True" w1785 {
                  tunnel: w1789 -> [_ w1793]
                  tunnel: w1788 -> [_ w1792]
                  tunnel: w1787 -> [_ w1791]
                  tunnel: w1786 -> [_ w1790]
                  frame False {
                  }
                  frame True {
                    n690 = Unbundle By Name(w1792) -> ("SET VALUE 10"=w1819:dbl, "TOL 10"=w1817:dbl, "RES VALUE 10"=w1815:dbl, "CH  PASS 10"=w1813:bool, "CH10 MAX TOL"=w1800:dbl, "CH10 MIN TOL"=w1799:dbl)
                    n691 = case shown="False" w1813 {
                      tunnel: ["FAIL" "PASS"] -> w1806
                      frame False {
                      }
                      frame True {
                      }
                    }
                    n692 = case shown="True" w1790 {
                      tunnel: ["NORMAL" "RETEST"] -> w1794
                      frame False {
                      }
                      frame True {
                      }
                    }
                    n693 = Get Date/Time String() -> (date string=w1811:string, time string=w1812:string)  [unwired: 3 in]
                    n694 = Concatenate Strings(w1811, w1812) -> (w1810:string)
                    n695 = Number To Fractional String(number=w1800, precision (6)=i16 3) -> (F-format string=w1798:string)  [unwired: 2 in]
                    n696 = Number To Fractional String(number=w1819, precision (6)=i16 3 ("width (-)")) -> (F-format string=w1809:string)  [unwired: 2 in]
                    n697 = Number To Fractional String(number=w1817, precision (6)=i16 3 ("width (-)")) -> (F-format string=w1808:string)  [unwired: 2 in]
                    n698 = Number To Fractional String(number=w1815, precision (6)=i16 3 ("width (-)")) -> (F-format string=w1807:string)  [unwired: 2 in]
                    n699 = Number To Fractional String(number=w1799, precision (6)=i16 3) -> (F-format string=w1797:string)  [unwired: 2 in]
                    n700 = Build Array(w1810, w1809, w1808, w1807, w1806, "10" ("element"), w1798, w1797, w1791, w1794) -> (w1804:string[])
                    n701 = call-poly <vilib>:"Write Delimited Spreadsheet.vi"("file path (dialog if empty)"=w1793, "1D data"=w1804, "append to file? (new file:F)"=TRUE, "transpose? (no:F)"=FALSE, "delimiter (\\t)"="," ("delimiter (\\t)")) -> ()  [unwired: 9 in, 2 out]
                  }
                }
              }
            }
          }
        }
      }
      frame "PART PRESENCE CHECKING" {
      }
    }
  }
